vi "new recipe file - Copy.vi"() -> ()   [LabVIEW 2018]
uses:
  <vilib>/Utility/file.llb/Read Delimited Spreadsheet (string).vi
panel:
  out "error out 2":errorcluster caption="error out"
  out "error out":errorcluster
  in  "hidden tab":enum32{"Page 1"}(tab)
  out "L dc length step 20":string
  out "L dc length step 19":string
  out "L dc length step 18":string
  out "L dc length step 17":string
  out "L dc length step 16":string
  out "L dc length step 15":string
  out "L dc length step 14":string
  out "L dc length step 13":string
  out "L dc length step 12":string
  out "L dc length step 11":string
  out "L dc power step 20":string
  out "L dc power step 19":string
  out "L dc power step 18":string
  out "L dc power step 17":string
  out "L dc power step 16":string
  out "L dc power step 15":string
  out "L dc power step 14":string
  out "L dc power step 13":string
  out "L dc power step 12":string
  out "L dc power step 11":string
  out "L pressure":string
  out "L argon flow":string
  out "L rf length step 10":string
  out "L rf length step 9":string
  out "L rf length step 8":string
  out "L rf length step 7":string
  out "L rf length step 6":string
  out "L rf length step 5":string
  out "L rf length step 4":string
  out "L rf length step 3":string
  out "L rf length step 2":string
  out "L rf length step 1":string
  out "L rf power step 10":string
  out "L rf power step 9":string
  out "L rf power step 8":string
  out "L rf power step 7":string
  out "L rf power step 6":string
  out "L rf power step 5":string
  out "L rf power step 4":string
  out "L rf power step 3":string
  out "L rf power step 2":string
  out "L rf power step 1":string
  out "L dc length step 10":string
  out "L dc length step 9":string
  out "L dc length step 8":string
  out "L dc length step 7":string
  out "L dc length step 6":string
  out "L dc length step 5":string
  out "L dc length step 4":string
  out "L dc length step 3":string
  out "L dc length step 2":string
  out "L dc length step 1":string
  out "L dc power step 10":string
  out "L dc power step 9":string
  out "L dc power step 8":string
  out "L dc power step 7":string
  out "L dc power step 6":string
  out "L dc power step 5":string
  out "L dc power step 4":string
  out "L dc power step 3":string
  out "L dc power step 2":string
  out "L dc power step 1":string
  out "L microwave power":string
  out "L chamber selection":string
  out "L single process type selection":string
  out "L tension  value":string
  out "L web speed":string
  out "L web thickness":string
  out "L left init diamater":string
  out "L core diamater":string
  out "L web selection":string
  out "L recipe selection":string
  out "L sbs name":string
  out "L recipe name":string
  out "total length error":bool
  out "left diameter after roll":dbl=8.0
  out "done":bool
  out "L dc step number":string
  out "L rf step number":string
  out "L rf length step 11":string
  out "L rf length step 12":string
  out "L rf length step 13":string
  out "L rf length step 14":string
  out "L rf length step 15":string
  out "L rf length step 16":string
  out "L rf length step 17":string
  out "L rf length step 18":string
  out "L rf length step 19":string
  out "L rf length step 20":string
  out "L rf power step 11":string
  out "L rf power step 12":string
  out "L rf power step 13":string
  out "L rf power step 14":string
  out "L rf power step 15":string
  out "L rf power step 16":string
  out "L rf power step 17":string
  out "L rf power step 18":string
  out "L rf power step 19":string
  out "L rf power step 20":string
  in  "steplist tab RF":enum32{"Page 1", "Page 2"}(tab)
  in  "rf step watt 20":dbl
  in  "rf step watt 19":dbl
  in  "rf step watt 18":dbl
  in  "rf step watt 17":dbl
  in  "rf step watt 16":dbl
  in  "rf step watt 15":dbl
  in  "rf step watt 14":dbl
  in  "rf step watt 13":dbl
  in  "rf step watt 12":dbl
  in  "rf step watt 11":dbl
  in  "rf step length 20":dbl
  in  "rf step length 19":dbl
  in  "rf step length 18":dbl
  in  "rf step length 17":dbl
  in  "rf step length 16":dbl
  in  "rf step length 15":dbl
  in  "rf step length 14":dbl
  in  "rf step length 13":dbl
  in  "rf step length 12":dbl
  in  "rf step length 11":dbl
  in  "rf step length 1":dbl
  in  "rf step length 2":dbl
  in  "rf step length 3":dbl
  in  "rf step length 4":dbl
  in  "rf step length 5":dbl
  in  "rf step length 6":dbl
  in  "rf step length 7":dbl
  in  "rf step length 8":dbl
  in  "rf step length 9":dbl
  in  "rf step length 10":dbl
  in  "rf step watt 1":dbl
  in  "rf step watt 2":dbl
  in  "rf step watt 3":dbl
  in  "rf step watt 4":dbl
  in  "rf step watt 7":dbl
  in  "rf step watt 8":dbl
  in  "rf step watt 5":dbl
  in  "rf step watt 6":dbl
  in  "rf step watt 9":dbl
  in  "rf step watt 10":dbl
  in  "Step Number RF":u16(ring) items=["step 1"=1, "step 2"=2, "step 3"=3, "step 4"=4, "step 5"=5, "step 6"=6, "step 7"=7, "step 8"=8, "step 9"=9, "step 10"=10, "step 11"=11, "step 12"=12, "step 13"=13, "step 14"=14, "step 15"=15, "step 16"=16, "step 17"=17, "step 18"=18, "step 19"=19, "step 20"=20]
  out "concatenated string":string
  in  "steplist tab DC":enum32{"Page 1", "Page 2"}(tab)
  in  "dc step watt 1":dbl
  in  "dc step watt 2":dbl
  in  "dc step watt 3":dbl
  in  "dc step watt 4":dbl
  in  "dc step watt 5":dbl
  in  "dc step watt 6":dbl
  in  "dc step watt 7":dbl
  in  "dc step watt 8":dbl
  in  "dc step watt 9":dbl
  in  "dc step watt 10":dbl
  in  "dc step length 1":dbl
  in  "dc step length 2":dbl
  in  "dc step length 3":dbl
  in  "dc step length 4":dbl
  in  "dc step length 5":dbl
  in  "dc step length 6":dbl
  in  "dc step length 7":dbl
  in  "dc step length 8":dbl
  in  "dc step length 9":dbl
  in  "dc step length 10":dbl
  in  "Step Number DC":u16(ring) items=["step 1"=1, "step 2"=2, "step 3"=3, "step 4"=4, "step 5"=5, "step 6"=6, "step 7"=7, "step 8"=8, "step 9"=9, "step 10"=10, "step 11"=11, "step 12"=12, "step 13"=13, "step 14"=14, "step 15"=15, "step 16"=16, "step 17"=17, "step 18"=18, "step 19"=19, "step 20"=20]
  in  "dc step watt 20":dbl
  in  "dc step watt 19":dbl
  in  "dc step watt 18":dbl
  in  "dc step watt 17":dbl
  in  "dc step watt 16":dbl
  in  "dc step watt 15":dbl
  in  "dc step watt 14":dbl
  in  "dc step watt 13":dbl
  in  "dc step watt 12":dbl
  in  "dc step watt 11":dbl
  in  "dc step length 11":dbl
  in  "dc step length 12":dbl
  in  "dc step length 13":dbl
  in  "dc step length 14":dbl
  in  "dc step length 15":dbl
  in  "dc step length 16":dbl
  in  "dc step length 17":dbl
  in  "dc step length 18":dbl
  in  "dc step length 19":dbl
  in  "dc step length 20":dbl
  in  "General tab sub vi":enum32{"Page 1"}(tab)
  in  "Pressure set mbar":dbl=0.005 format="%#_1e"
  in  "Ar set sccm":dbl=20.0
  in  "CANCEL":bool
  in  "SAVE":bool
  in  "web-other tab":T1(tab)
  out "total length":dbl=500.0
  in  "tension value":dbl=7.0
  in  "web speed":dbl=250.0
  in  "web thickness":dbl=50.0
  in  "left initial diameter":dbl=94.0
  in  "core diameter":dbl=93.0
  in  "CALCULATE":bool
  in  "Web Selection":u16(ring) items=["web", "other"]
  in  "Recipe Selection":u16(ring) items=["single recipe", "multilayer recipe"]
  in  "Recipe Name":string
  in  "Substrate Material":string
  in  "recipe selection":T2(tab)
  in  "single process selection":enum32{"microwave", "dcsputter", "rfsputter"}(radio)
  in  "single process selection":T3(tab)
  in  "power microwave":dbl
  in  "DC Sputter Chamber Selection":enum32{"chamber II", "chamber III"}(radio)
  in  "power rf":dbl
  in  "web speed ch III ml":dbl=250.0
  in  "web speed ch II ml":dbl=250.0
  in  "LOAD":bool
  in  "password":bool
  in  "password":string
  # "Step List(RF)"
  # "power(watt)"
  # "length(cm)"
  # "Step 1"
  # "Step 2"
  # "Step 3"
  # "Step 4"
  # "Step 5"
  # "Step 6"
  # "Step 7"
  # "Step 8"
  # "Step 9"
  # "Step 10"
  # "Step 11"
  # "Step 12"
  # "Step 13"
  # "Step 14"
  # "Step 15"
  # "Step 16"
  # "Step 17"
  # "Step 18"
  # "Step 19"
  # "Step 20"
  # "Step List(DC)"
  # "power(watt)"
  # "length(cm)"
  # "Step 1"
  # "Step 2"
  # "Step 3"
  # "Step 4"
  # "Step 5"
  # "Step 6"
  # "Step 7"
  # "Step 8"
  # "Step 9"
  # "Step 10"
  # "Step 11"
  # "Step 12"
  # "Step 13"
  # "Step 14"
  # "Step 15"
  # "Step 16"
  # "Step 17"
  # "Step 18"
  # "Step 19"
  # "Step 20"
  # "Recipe Name"
  # "Subsrate Material"
  # "Recipe Selection"
  # "Web Selection"
  # "Argon Flow"
  # "sccm"
  # "Set Pressure"
  # "mbar"
  # "Core Diameter"
  # "mm"
  # "Web Speed"
  # "cm/min"
  # "Left InitialDiameter"
  # "mm"
  # "Tension Value"
  # "N"
  # "µm"
  # "cm"
  # "Web Thickness"
  # "Total Length"
  # "Power"
  # "watt"
  # "Power"
  # "watt"
  # "DCPS PARAMETERS"
  # "Chamber III"
  # "Chamber II"
  # "Web Speed"
  # "cm/min"
  # "Web Speed"
  # "cm/min"
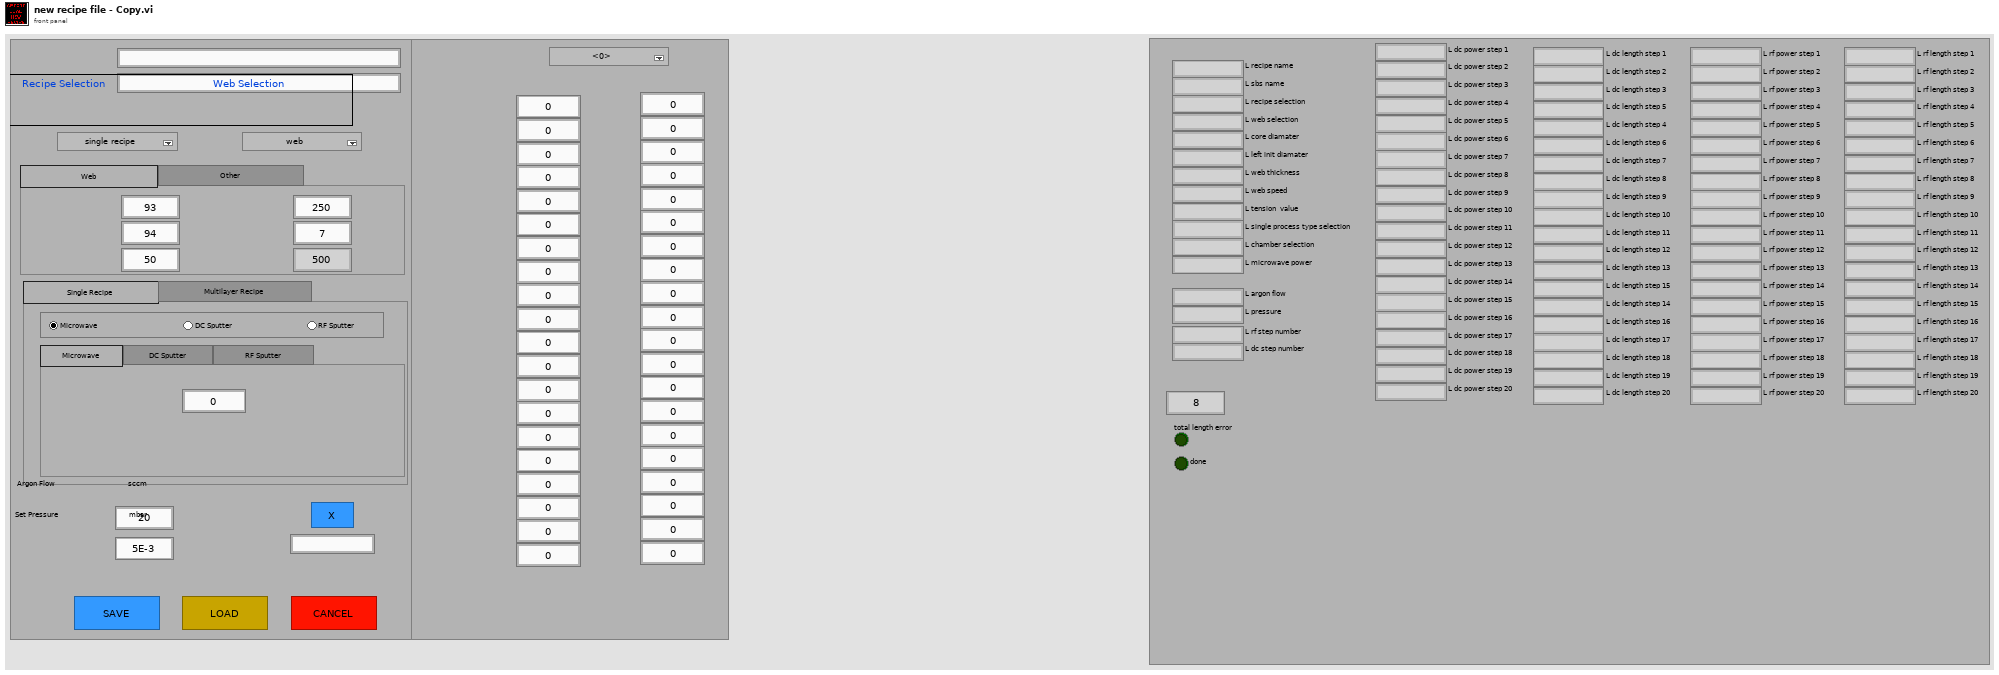
[diagram p1: front panel]
types:
  T1 = enum32{"Web                                                    ", "Other                                                      "}
  T2 = enum32{"Single Recipe                                    ", "Multilayer Recipe                                      "}
  T3 = enum32{"Microwave                ", "DC Sputter                   ", "RF Sputter                         "}
  T4 = enum16{"open", "replace", "create", "open or create", "replace or create", "replace or create with confirmation"}
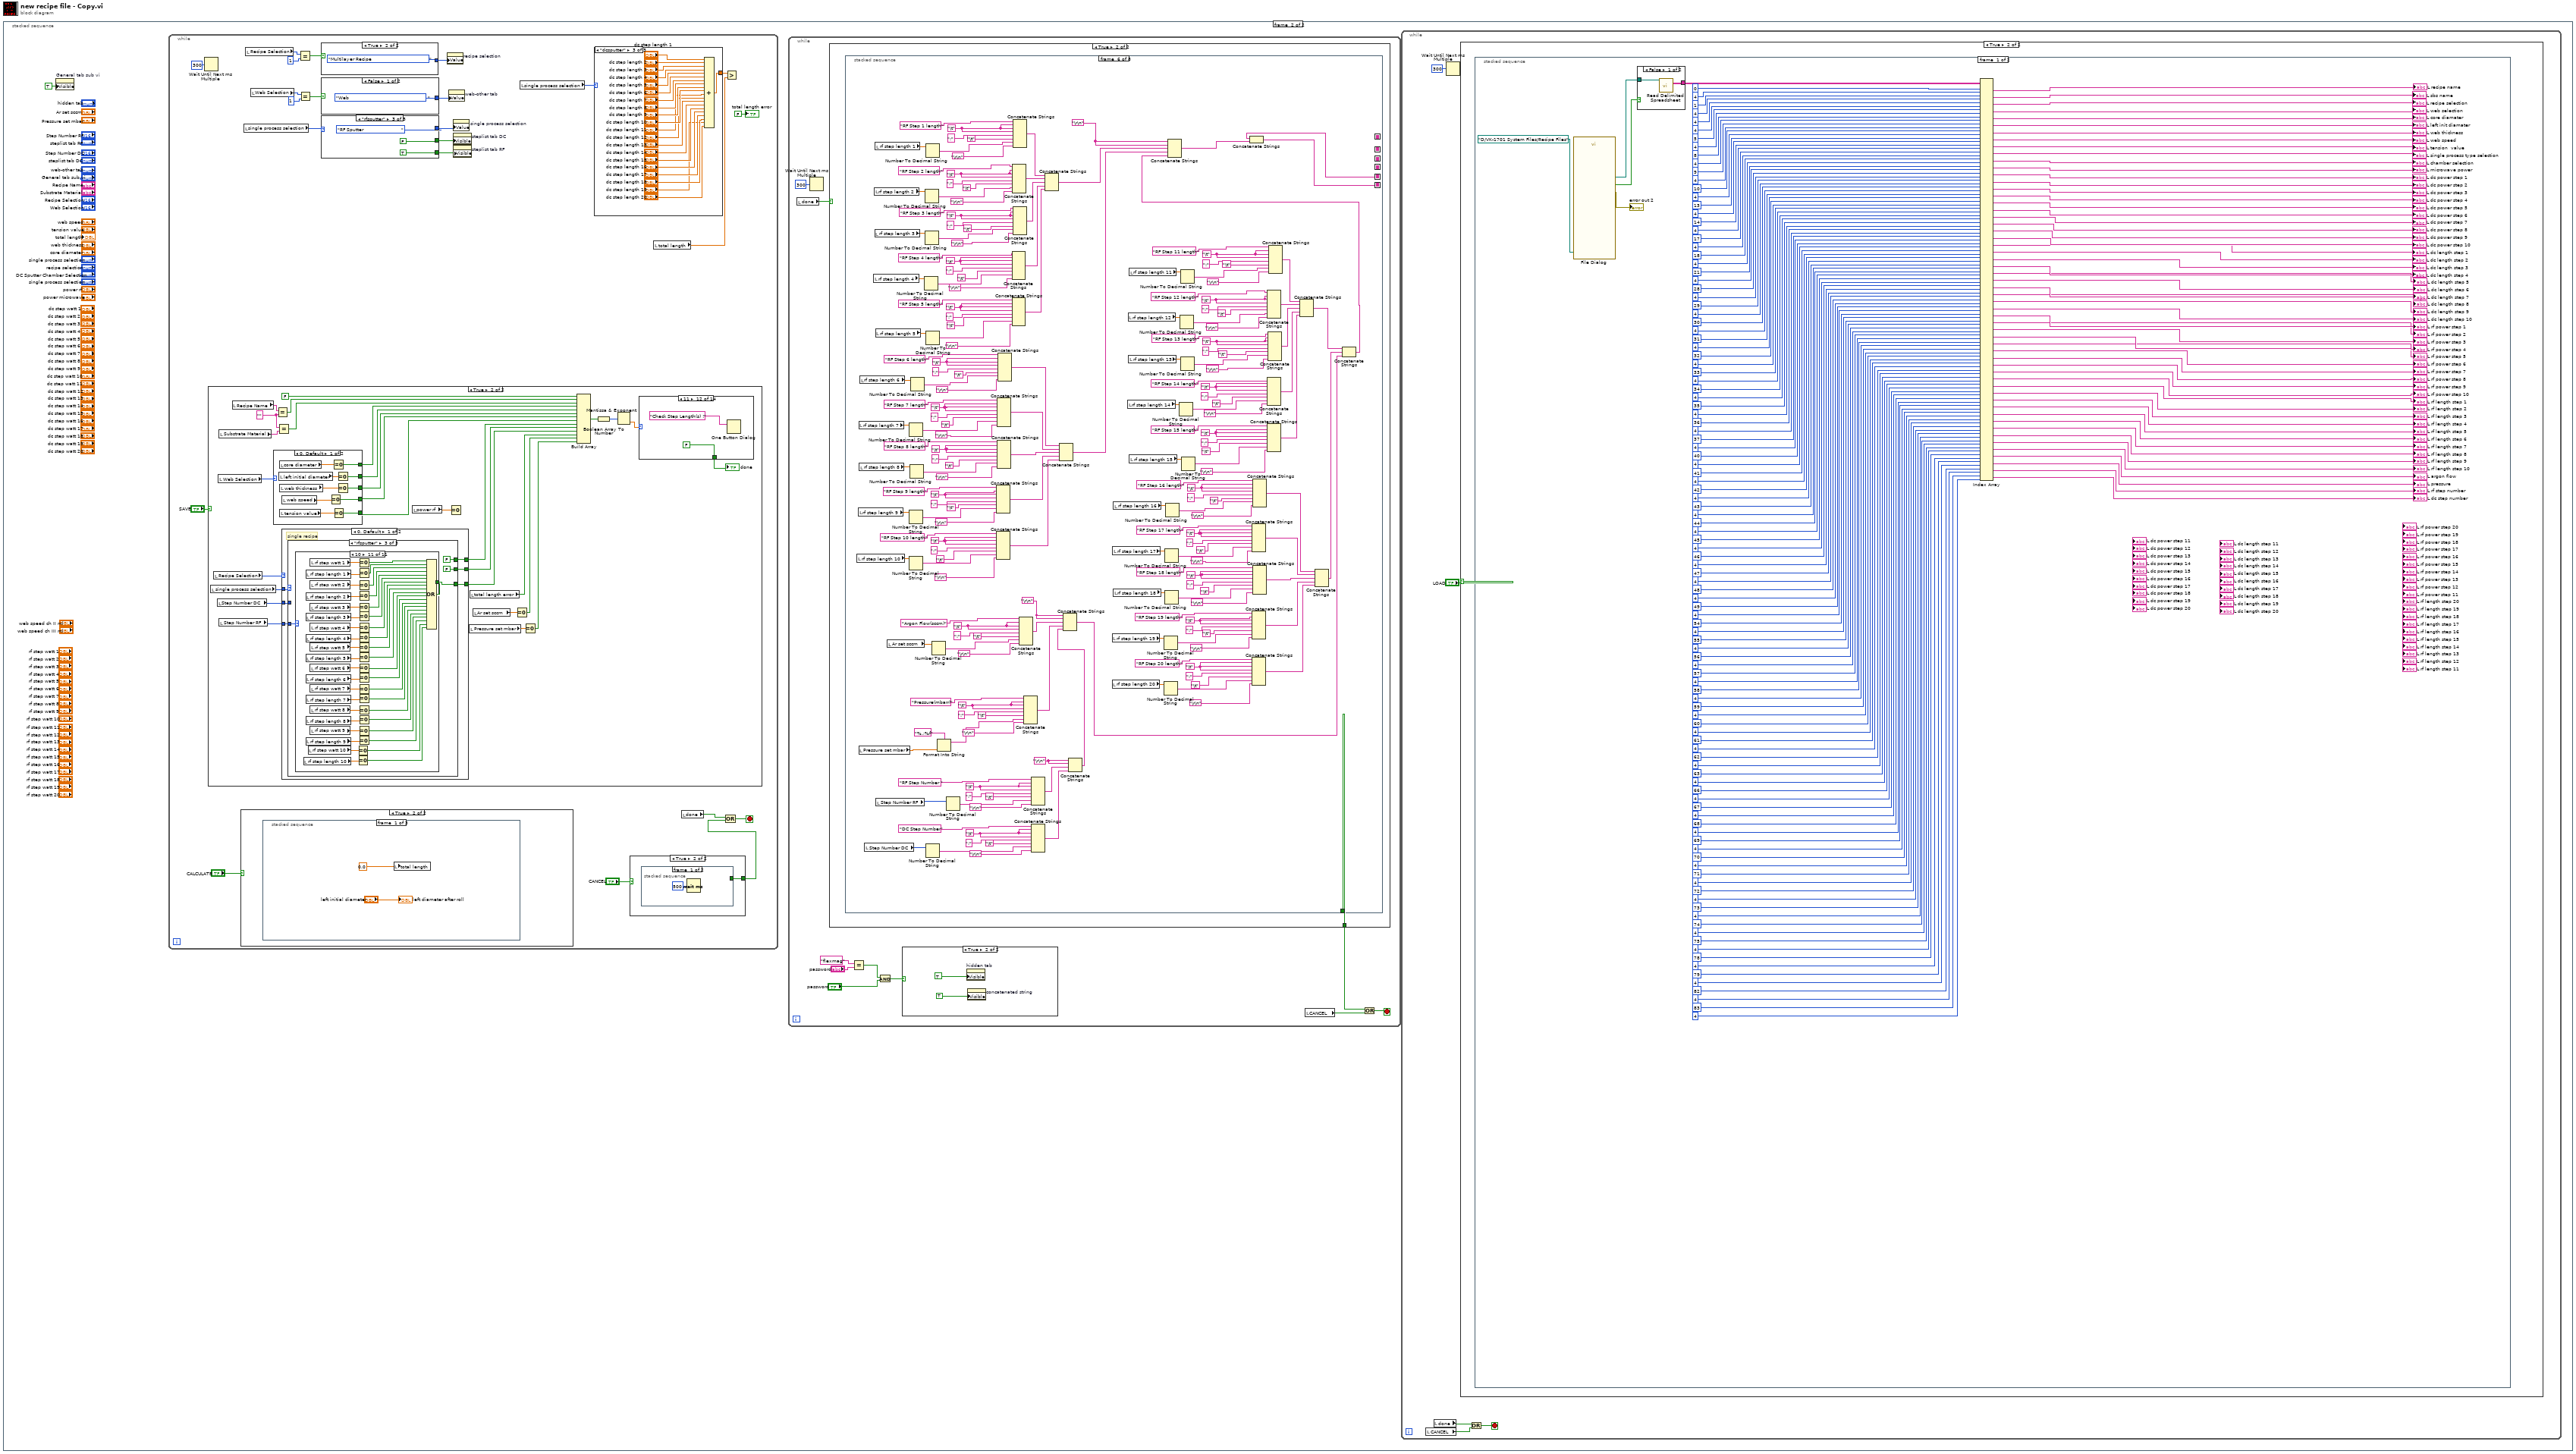
[diagram p0: block diagram]
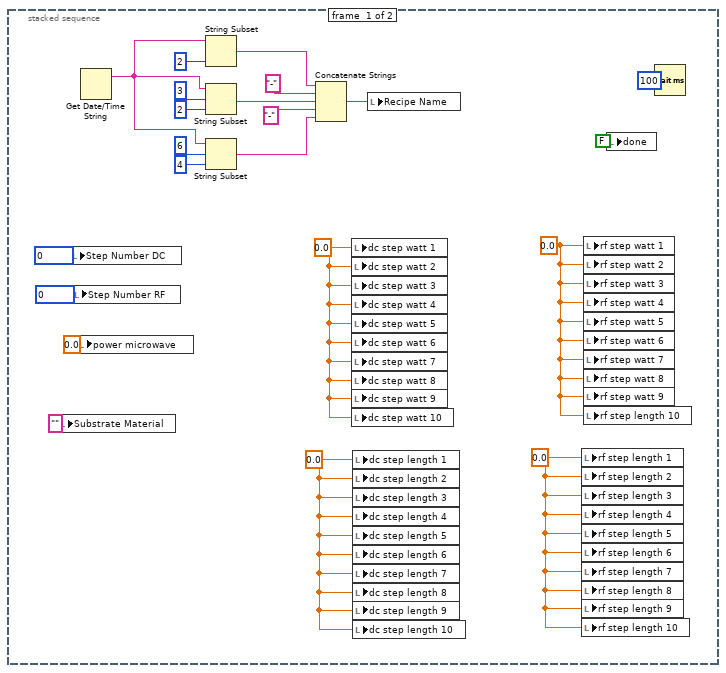
[diagram p2: hidden frame]
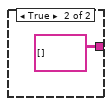
[diagram p4: hidden frame]
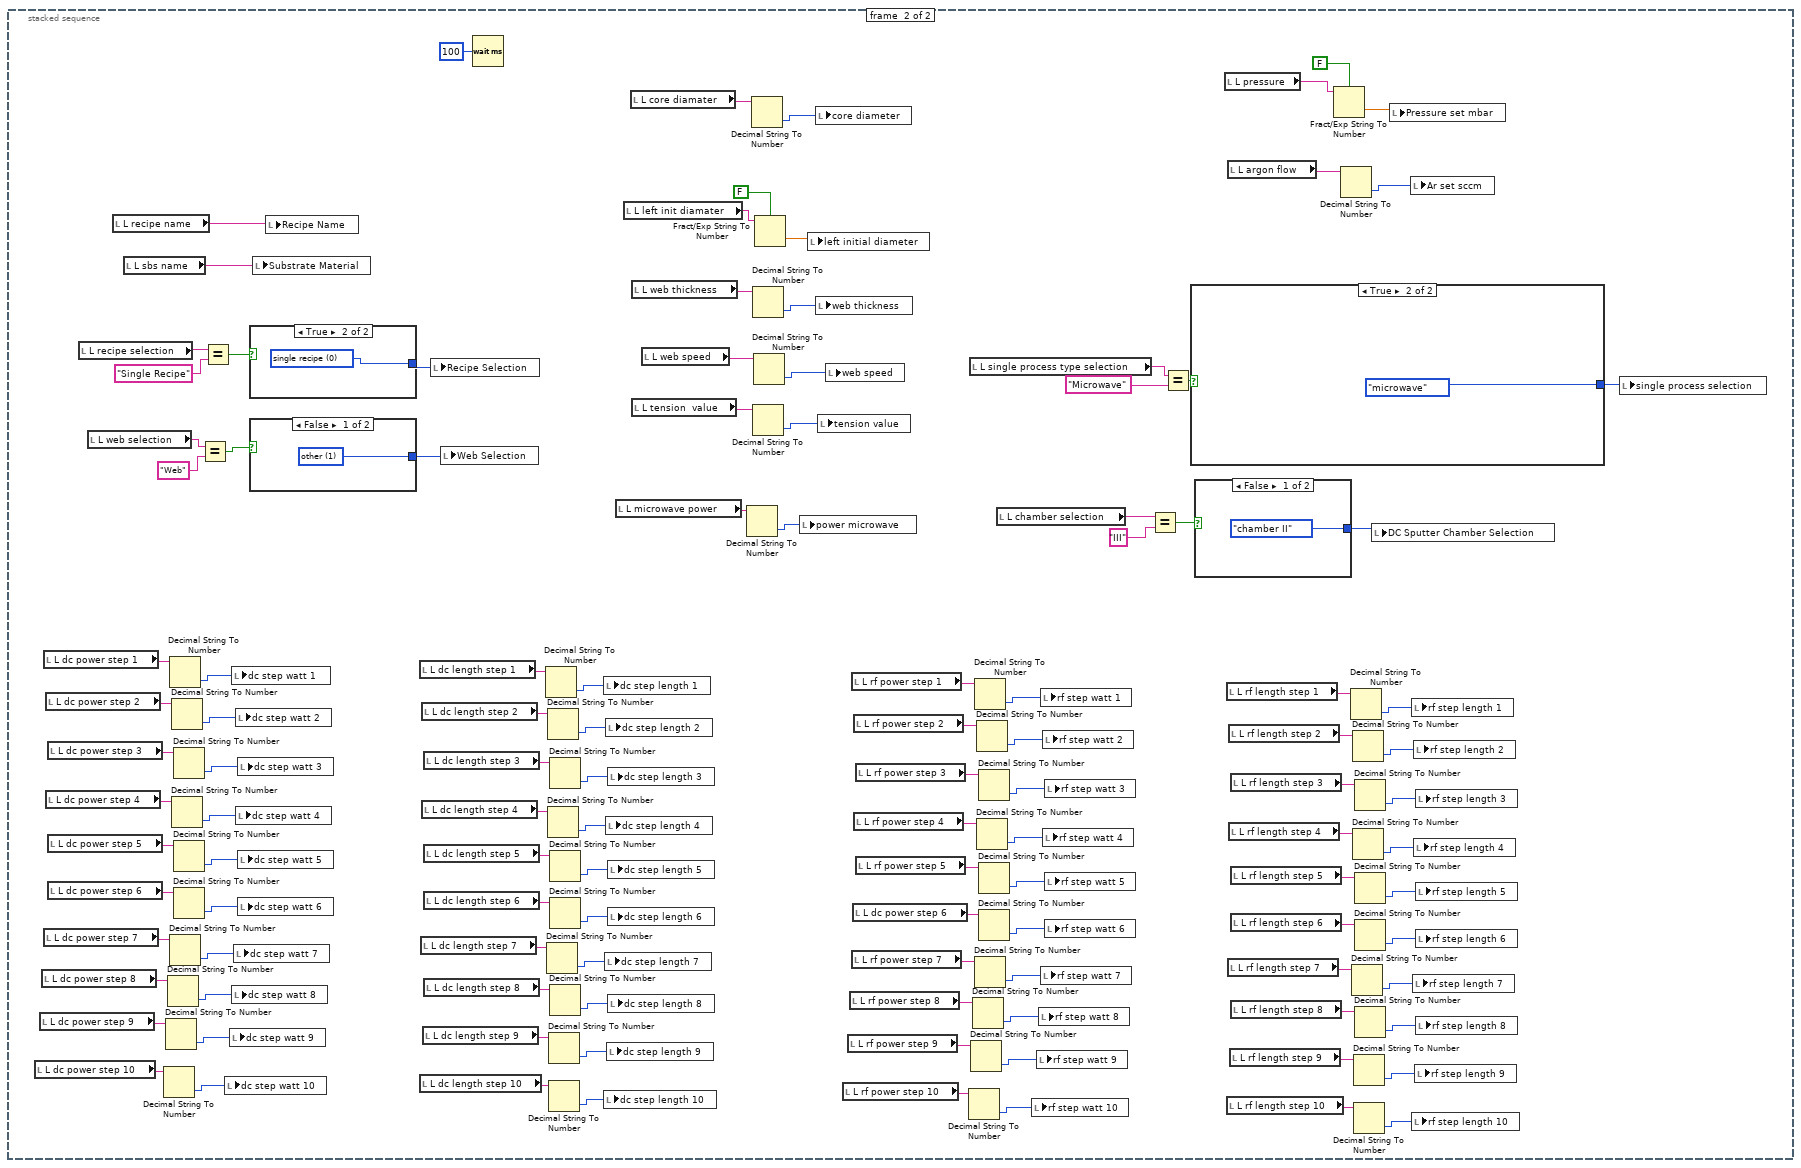
[diagram p5: hidden frame]
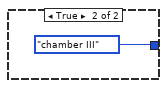
[diagram p6: hidden frame]
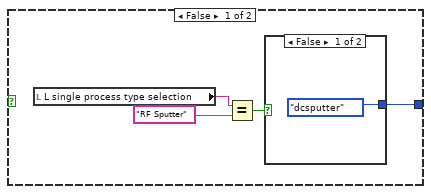
[diagram p7: hidden frame]
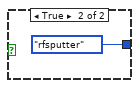
[diagram p8: hidden frame]
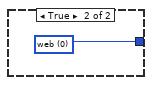
[diagram p9: hidden frame]
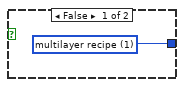
[diagram p10: hidden frame]
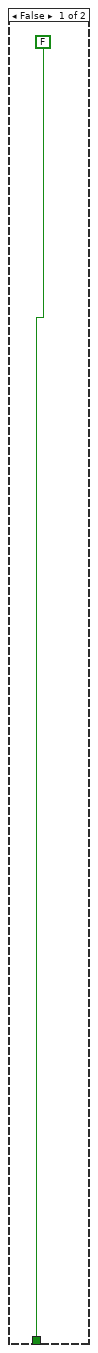
[diagram p12: hidden frame]
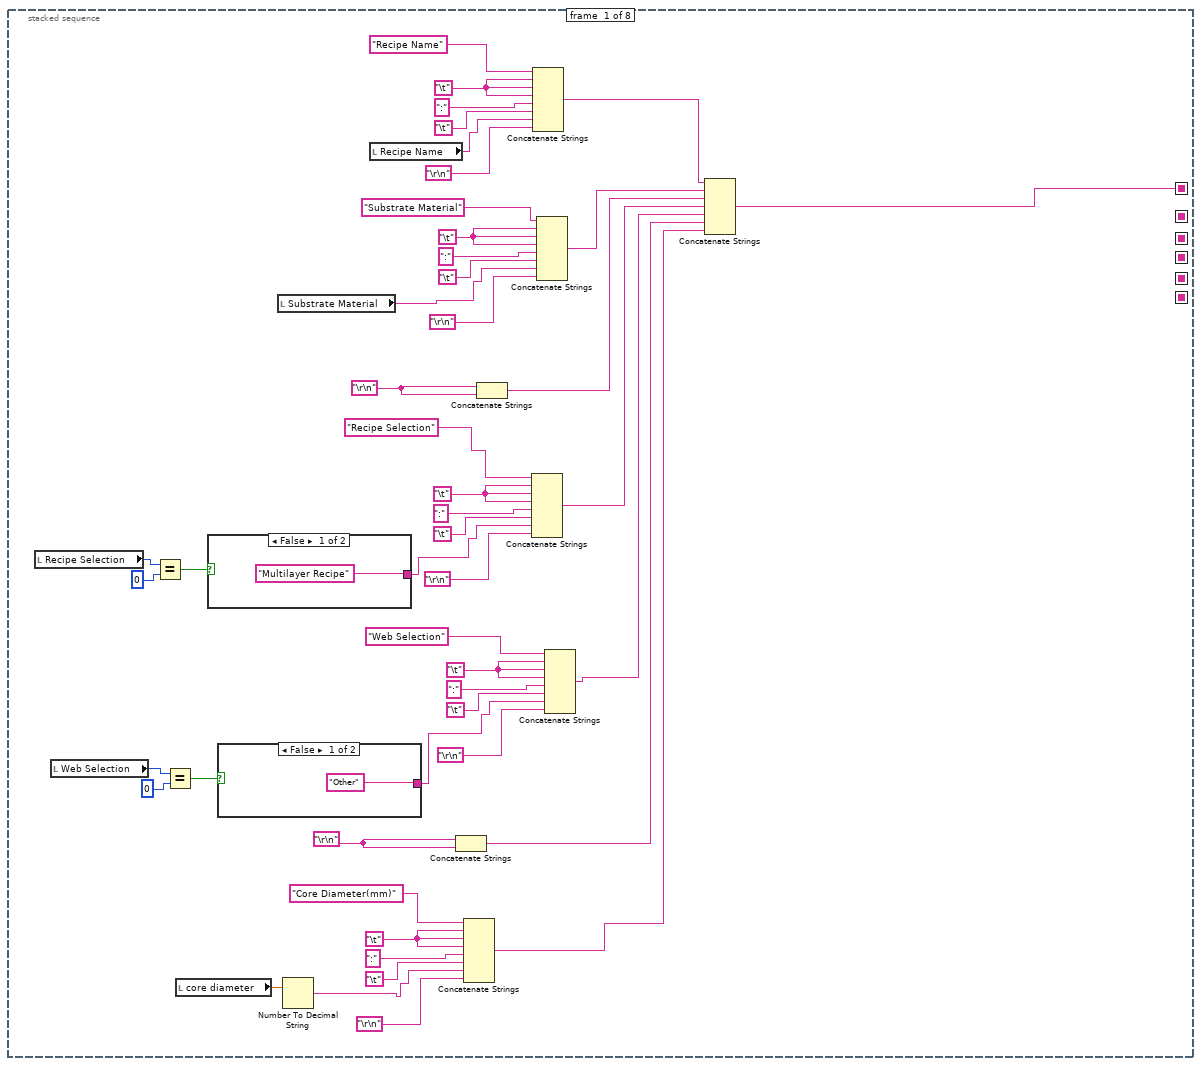
[diagram p13: hidden frame]
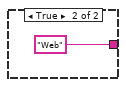
[diagram p14: hidden frame]
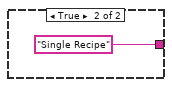
[diagram p15: hidden frame]
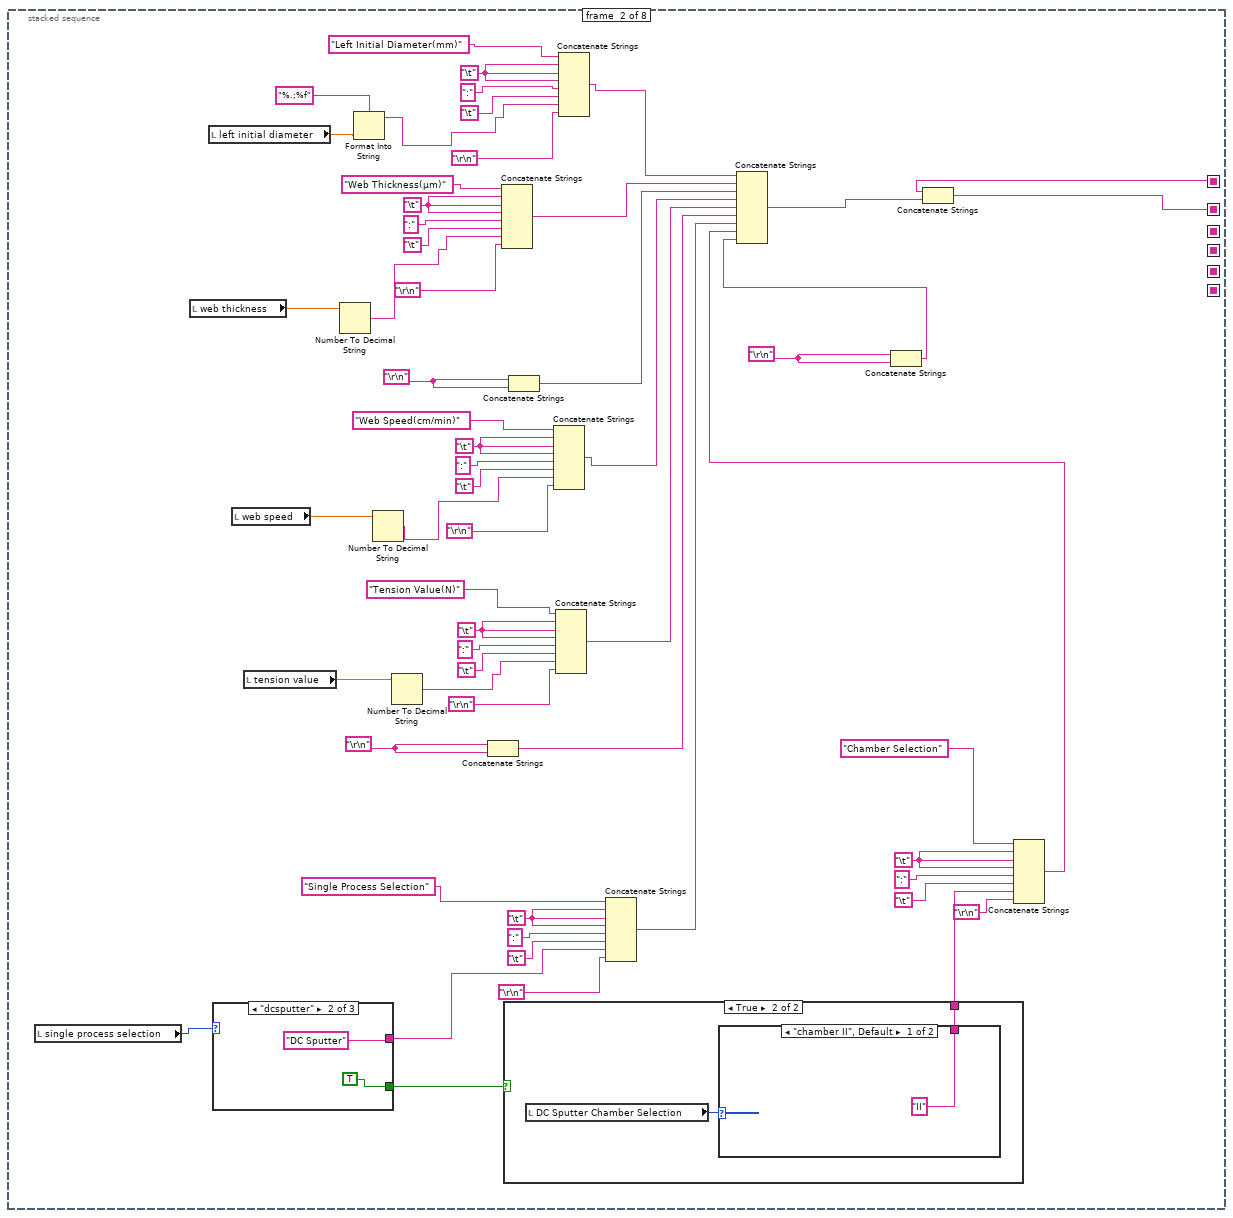
[diagram p16: hidden frame]
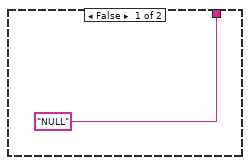
[diagram p17: hidden frame]
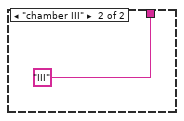
[diagram p18: hidden frame]
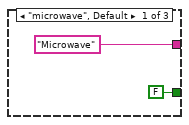
[diagram p19: hidden frame]
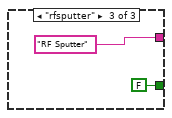
[diagram p20: hidden frame]
diagram:
  n1 = stacked-sequence {
    frame #0 {
      w3 = u16 0 items=["step 1"=1, "step 2"=2, "step 3"=3, "step 4"=4, "step 5"=5, "step 6"=6, "step 7"=7, "step 8"=8, "step 9"=9, "step 10"=10] ("Step Number DC")
      w5 = 0.0 ("dc step watt 1")
      w4 = 0.0 ("dc step watt 1")
      w6 = u16 0 items=["step 1"=1, "step 2"=2, "step 3"=3, "step 4"=4, "step 5"=5, "step 6"=6, "step 7"=7, "step 8"=8, "step 9"=9, "step 10"=10] ("Step Number DC")
      w7 = 0.0 ("dc step watt 1")
      w8 = 0.0 ("dc step watt 1")
      n2 = local write "Substrate Material"("" ("Substrate Material")) -> ()
      n3 = local write "Step Number DC"(w6) -> ()
      n4 = local write "Step Number RF"(w3) -> ()
      n5 = local write "power microwave"(0.0 ("power microwave")) -> ()
      n6 = Get Date/Time String() -> (date string=w16:string)  [unwired: 3 in, 1 out]
      n7 = String Subset(string=w16, length (rest)=2 ("length (rest)")) -> (substring=w17:string)  [unwired: 1 in]
      n8 = String Subset(string=w16, offset (0)=3, length (rest)=2 ("length (rest)")) -> (substring=w18:string)
      n9 = String Subset(string=w16, offset (0)=6, length (rest)=4 ("length (rest)")) -> (substring=w19:string)
      n10 = Concatenate Strings(w17, "-" ("string"), w18, "-" ("string"), w19) -> (w20:string)
      n11 = local write "dc step watt 1"(w8) -> ()
      n12 = local write "dc step watt 2"(w8) -> ()
      n13 = local write "dc step watt 3"(w8) -> ()
      n14 = local write "dc step watt 4"(w8) -> ()
      n15 = local write "dc step watt 5"(w8) -> ()
      n16 = local write "dc step watt 6"(w8) -> ()
      n17 = local write "dc step watt 7"(w8) -> ()
      n18 = local write "dc step watt 8"(w8) -> ()
      n19 = local write "dc step watt 9"(w8) -> ()
      n20 = local write "dc step watt 10"(w8) -> ()
      n21 = local write "dc step length 1"(w7) -> ()
      n22 = local write "dc step length 2"(w7) -> ()
      n23 = local write "dc step length 3"(w7) -> ()
      n24 = local write "dc step length 4"(w7) -> ()
      n25 = local write "dc step length 5"(w7) -> ()
      n26 = local write "dc step length 6"(w7) -> ()
      n27 = local write "dc step length 7"(w7) -> ()
      n28 = local write "dc step length 8"(w7) -> ()
      n29 = local write "dc step length 9"(w7) -> ()
      n30 = local write "dc step length 10"(w7) -> ()
      n31 = local write "Recipe Name"(w20) -> ()
      n32 = local write "rf step length 1"(w5) -> ()
      n33 = local write "rf step length 2"(w5) -> ()
      n34 = local write "rf step length 3"(w5) -> ()
      n35 = local write "rf step length 4"(w5) -> ()
      n36 = local write "rf step length 5"(w5) -> ()
      n37 = local write "rf step length 6"(w5) -> ()
      n38 = local write "rf step length 7"(w5) -> ()
      n39 = local write "rf step length 8"(w5) -> ()
      n40 = local write "rf step length 9"(w5) -> ()
      n41 = local write "rf step length 10"(w5) -> ()
      n42 = local write "rf step watt 1"(w4) -> ()
      n43 = local write "rf step watt 2"(w4) -> ()
      n44 = local write "rf step watt 3"(w4) -> ()
      n45 = local write "rf step watt 4"(w4) -> ()
      n46 = local write "rf step watt 5"(w4) -> ()
      n47 = local write "rf step watt 6"(w4) -> ()
      n48 = local write "rf step watt 7"(w4) -> ()
      n49 = local write "rf step watt 8"(w4) -> ()
      n50 = local write "rf step watt 9"(w4) -> ()
      n51 = local write "rf step length 10"(w4) -> ()
      n52 = local write "done"(FALSE ("done")) -> ()
      n53 = Wait (ms)(milliseconds to wait=u32 100) -> ()  [unwired: 1 out]
    }
    frame #1 {
      n54 = property on="General tab sub vi" class="TabCtl (strict)"("Visible"=TRUE) -> ()  [unwired: 2 in, 2 out]
      n55 = while {
        stop <- w1227 stop-if-true
        n56 = Wait Until Next ms Multiple(millisecond multiple=u32 300) -> ()  [unwired: 1 out]
        n57 = case shown="True" "SAVE" {
          frame False {
          }
          frame True {
            w1345 = "" ("y")
            n58 = local read "single process selection"() -> (w1331:enum32{"microwave", "dcsputter", "rfsputter"})
            n59 = local read "Recipe Selection"() -> (w1332:u16)
            n60 = local read "Step Number DC"() -> (w1330:u16)
            n61 = local read "Web Selection"() -> (w1339:u16)
            n62 = local read "Substrate Material"() -> (w1346:string)
            n63 = local read "Step Number RF"() -> (w1319:u16)
            n64 = local read "Recipe Name"() -> (w1347:string)
            n65 = case shown="0, Default" w1339 {
              tunnel: [w1836 w1841] -> w1338
              tunnel: [w1835 w1841] -> w1337
              tunnel: [w1834 w1841] -> w1336
              tunnel: [w1833 w1841] -> w1334
              tunnel: [w1831 w1841] -> w1335
              frame 0, Default {
                n66 = local read "left initial diameter"() -> (w1839:dbl)
                n67 = local read "core diameter"() -> (w1840:dbl)
                n68 = local read "web thickness"() -> (w1838:dbl)
                n69 = local read "tension value"() -> (w1837:dbl)
                n70 = local read "web speed"() -> (w1832:dbl)
                n71 = Equal To 0?(x=w1832) -> (x = 0?=w1831:bool)
                n72 = Equal To 0?(x=w1840) -> (x = 0?=w1836:bool)
                n73 = Equal To 0?(x=w1837) -> (x = 0?=w1833:bool)
                n74 = Equal To 0?(x=w1839) -> (x = 0?=w1835:bool)
                n75 = Equal To 0?(x=w1838) -> (x = 0?=w1834:bool)
              }
              frame 1 {
                w1841 = FALSE
              }
            }
            n76 = Equal?(x=w1347, y=w1345) -> (x = y?=w1341:bool)
            n77 = Equal?(x=w1345, y=w1346) -> (x = y?=w1340:bool)
            n78 = case shown="0, Default" w1332 {
              tunnel: w1331 -> [w1353 _]
              tunnel: w1330 -> [w1352 _]
              tunnel: [w1351 FALSE] -> w1329
              tunnel: [w1350 FALSE] -> w1328
              tunnel: [w1349 FALSE] -> w1327
              tunnel: w1319 -> [w1348 _]
              frame 0, Default {
                # "single recipe"
                n79 = case shown="\"rfsputter\"" w1353 {
                  tunnel: w1352 -> [_ w1361 _]
                  tunnel: [w1356 FALSE FALSE] -> w1351
                  tunnel: [FALSE w1360 FALSE] -> w1350
                  tunnel: [FALSE FALSE w1594] -> w1349
                  tunnel: w1348 -> [_ _ w1593]
                  frame "microwave", Default {
                    n80 = local read "power microwave"() -> (w1357:dbl)
                    n81 = Equal To 0?(x=w1357) -> (x = 0?=w1356:bool)
                  }
                  frame "dcsputter" {
                    n82 = case shown="1" w1361 {
                      tunnel: [FALSE w1363 w1372 w1385 w1402 w1423 w1448 w1477 w1510 w1547 w1588] -> w1360
                      frame 0, Default {
                      }
                      frame 1 {
                        n83 = local read "dc step length 1"() -> (w1366:dbl)
                        n84 = local read "dc step watt 1"() -> (w1367:dbl)
                        n85 = Equal To 0?(x=w1367) -> (x = 0?=w1365:bool)
                        n86 = Equal To 0?(x=w1366) -> (x = 0?=w1364:bool)
                        n87 = Compound Arithmetic op=OR(w1365, w1364) -> (w1363:bool)
                      }
                      frame 2 {
                        n88 = local read "dc step length 1"() -> (w1375:dbl)
                        n89 = local read "dc step length 2"() -> (w1371:dbl)
                        n90 = local read "dc step watt 1"() -> (w1376:dbl)
                        n91 = local read "dc step watt 2"() -> (w1370:dbl)
                        n92 = Equal To 0?(x=w1376) -> (x = 0?=w1374:bool)
                        n93 = Equal To 0?(x=w1370) -> (x = 0?=w1369:bool)
                        n94 = Equal To 0?(x=w1375) -> (x = 0?=w1373:bool)
                        n95 = Equal To 0?(x=w1371) -> (x = 0?=w1368:bool)
                        n96 = Compound Arithmetic op=OR(w1374, w1373, w1369, w1368) -> (w1372:bool)
                      }
                      frame 3 {
                        n97 = local read "dc step length 1"() -> (w1388:dbl)
                        n98 = local read "dc step length 2"() -> (w1384:dbl)
                        n99 = local read "dc step length 3"() -> (w1379:dbl)
                        n100 = local read "dc step watt 1"() -> (w1389:dbl)
                        n101 = local read "dc step watt 2"() -> (w1383:dbl)
                        n102 = local read "dc step watt 3"() -> (w1380:dbl)
                        n103 = Equal To 0?(x=w1389) -> (x = 0?=w1387:bool)
                        n104 = Equal To 0?(x=w1383) -> (x = 0?=w1382:bool)
                        n105 = Equal To 0?(x=w1388) -> (x = 0?=w1386:bool)
                        n106 = Equal To 0?(x=w1380) -> (x = 0?=w1378:bool)
                        n107 = Equal To 0?(x=w1384) -> (x = 0?=w1381:bool)
                        n108 = Equal To 0?(x=w1379) -> (x = 0?=w1377:bool)
                        n109 = Compound Arithmetic op=OR(w1387, w1386, w1382, w1381, w1378, w1377) -> (w1385:bool)
                      }
                      frame 4 {
                        n110 = local read "dc step length 1"() -> (w1405:dbl)
                        n111 = local read "dc step length 4"() -> (w1393:dbl)
                        n112 = local read "dc step length 2"() -> (w1401:dbl)
                        n113 = local read "dc step length 3"() -> (w1396:dbl)
                        n114 = local read "dc step watt 1"() -> (w1406:dbl)
                        n115 = local read "dc step watt 2"() -> (w1400:dbl)
                        n116 = local read "dc step watt 4"() -> (w1392:dbl)
                        n117 = local read "dc step watt 3"() -> (w1397:dbl)
                        n118 = Equal To 0?(x=w1406) -> (x = 0?=w1404:bool)
                        n119 = Equal To 0?(x=w1400) -> (x = 0?=w1399:bool)
                        n120 = Equal To 0?(x=w1392) -> (x = 0?=w1391:bool)
                        n121 = Equal To 0?(x=w1405) -> (x = 0?=w1403:bool)
                        n122 = Equal To 0?(x=w1397) -> (x = 0?=w1395:bool)
                        n123 = Equal To 0?(x=w1393) -> (x = 0?=w1390:bool)
                        n124 = Equal To 0?(x=w1401) -> (x = 0?=w1398:bool)
                        n125 = Equal To 0?(x=w1396) -> (x = 0?=w1394:bool)
                        n126 = Compound Arithmetic op=OR(w1404, w1403, w1399, w1398, w1395, w1394, w1391, w1390) -> (w1402:bool)
                      }
                      frame 5 {
                        n127 = local read "dc step length 5"() -> (w1409:dbl)
                        n128 = local read "dc step length 1"() -> (w1426:dbl)
                        n129 = local read "dc step length 4"() -> (w1414:dbl)
                        n130 = local read "dc step length 2"() -> (w1422:dbl)
                        n131 = local read "dc step length 3"() -> (w1417:dbl)
                        n132 = local read "dc step watt 1"() -> (w1427:dbl)
                        n133 = local read "dc step watt 5"() -> (w1410:dbl)
                        n134 = local read "dc step watt 2"() -> (w1421:dbl)
                        n135 = local read "dc step watt 4"() -> (w1413:dbl)
                        n136 = local read "dc step watt 3"() -> (w1418:dbl)
                        n137 = Equal To 0?(x=w1410) -> (x = 0?=w1408:bool)
                        n138 = Equal To 0?(x=w1427) -> (x = 0?=w1425:bool)
                        n139 = Equal To 0?(x=w1409) -> (x = 0?=w1407:bool)
                        n140 = Equal To 0?(x=w1421) -> (x = 0?=w1420:bool)
                        n141 = Equal To 0?(x=w1413) -> (x = 0?=w1412:bool)
                        n142 = Equal To 0?(x=w1426) -> (x = 0?=w1424:bool)
                        n143 = Equal To 0?(x=w1418) -> (x = 0?=w1416:bool)
                        n144 = Equal To 0?(x=w1414) -> (x = 0?=w1411:bool)
                        n145 = Equal To 0?(x=w1422) -> (x = 0?=w1419:bool)
                        n146 = Equal To 0?(x=w1417) -> (x = 0?=w1415:bool)
                        n147 = Compound Arithmetic op=OR(w1425, w1424, w1420, w1419, w1416, w1415, w1412, w1411, w1408, w1407) -> (w1423:bool)
                      }
                      frame 6 {
                        n148 = local read "dc step length 6"() -> (w1431:dbl)
                        n149 = local read "dc step length 5"() -> (w1434:dbl)
                        n150 = local read "dc step length 1"() -> (w1451:dbl)
                        n151 = local read "dc step length 4"() -> (w1439:dbl)
                        n152 = local read "dc step length 2"() -> (w1447:dbl)
                        n153 = local read "dc step length 3"() -> (w1442:dbl)
                        n154 = local read "dc step watt 6"() -> (w1430:dbl)
                        n155 = local read "dc step watt 1"() -> (w1452:dbl)
                        n156 = local read "dc step watt 5"() -> (w1435:dbl)
                        n157 = local read "dc step watt 2"() -> (w1446:dbl)
                        n158 = local read "dc step watt 4"() -> (w1438:dbl)
                        n159 = local read "dc step watt 3"() -> (w1443:dbl)
                        n160 = Equal To 0?(x=w1430) -> (x = 0?=w1429:bool)
                        n161 = Equal To 0?(x=w1431) -> (x = 0?=w1428:bool)
                        n162 = Equal To 0?(x=w1435) -> (x = 0?=w1433:bool)
                        n163 = Equal To 0?(x=w1452) -> (x = 0?=w1450:bool)
                        n164 = Equal To 0?(x=w1434) -> (x = 0?=w1432:bool)
                        n165 = Equal To 0?(x=w1446) -> (x = 0?=w1445:bool)
                        n166 = Equal To 0?(x=w1438) -> (x = 0?=w1437:bool)
                        n167 = Equal To 0?(x=w1451) -> (x = 0?=w1449:bool)
                        n168 = Equal To 0?(x=w1443) -> (x = 0?=w1441:bool)
                        n169 = Equal To 0?(x=w1439) -> (x = 0?=w1436:bool)
                        n170 = Equal To 0?(x=w1447) -> (x = 0?=w1444:bool)
                        n171 = Equal To 0?(x=w1442) -> (x = 0?=w1440:bool)
                        n172 = Compound Arithmetic op=OR(w1450, w1449, w1445, w1444, w1441, w1440, w1437, w1436, w1433, w1432, w1429, w1428) -> (w1448:bool)
                      }
                      frame 7 {
                        n173 = local read "dc step length 6"() -> (w1460:dbl)
                        n174 = local read "dc step length 7"() -> (w1455:dbl)
                        n175 = local read "dc step length 5"() -> (w1463:dbl)
                        n176 = local read "dc step length 1"() -> (w1480:dbl)
                        n177 = local read "dc step length 4"() -> (w1468:dbl)
                        n178 = local read "dc step length 2"() -> (w1476:dbl)
                        n179 = local read "dc step length 3"() -> (w1471:dbl)
                        n180 = local read "dc step watt 6"() -> (w1459:dbl)
                        n181 = local read "dc step watt 7"() -> (w1456:dbl)
                        n182 = local read "dc step watt 1"() -> (w1481:dbl)
                        n183 = local read "dc step watt 5"() -> (w1464:dbl)
                        n184 = local read "dc step watt 2"() -> (w1475:dbl)
                        n185 = local read "dc step watt 4"() -> (w1467:dbl)
                        n186 = local read "dc step watt 3"() -> (w1472:dbl)
                        n187 = Equal To 0?(x=w1459) -> (x = 0?=w1458:bool)
                        n188 = Equal To 0?(x=w1456) -> (x = 0?=w1454:bool)
                        n189 = Equal To 0?(x=w1460) -> (x = 0?=w1457:bool)
                        n190 = Equal To 0?(x=w1455) -> (x = 0?=w1453:bool)
                        n191 = Equal To 0?(x=w1464) -> (x = 0?=w1462:bool)
                        n192 = Equal To 0?(x=w1481) -> (x = 0?=w1479:bool)
                        n193 = Equal To 0?(x=w1463) -> (x = 0?=w1461:bool)
                        n194 = Equal To 0?(x=w1475) -> (x = 0?=w1474:bool)
                        n195 = Equal To 0?(x=w1467) -> (x = 0?=w1466:bool)
                        n196 = Equal To 0?(x=w1480) -> (x = 0?=w1478:bool)
                        n197 = Equal To 0?(x=w1472) -> (x = 0?=w1470:bool)
                        n198 = Equal To 0?(x=w1468) -> (x = 0?=w1465:bool)
                        n199 = Equal To 0?(x=w1476) -> (x = 0?=w1473:bool)
                        n200 = Equal To 0?(x=w1471) -> (x = 0?=w1469:bool)
                        n201 = Compound Arithmetic op=OR(w1479, w1478, w1474, w1473, w1470, w1469, w1466, w1465, w1462, w1461, w1458, w1457, w1454, w1453) -> (w1477:bool)
                      }
                      frame 8 {
                        n202 = local read "dc step length 6"() -> (w1493:dbl)
                        n203 = local read "dc step length 7"() -> (w1488:dbl)
                        n204 = local read "dc step length 8"() -> (w1485:dbl)
                        n205 = local read "dc step length 5"() -> (w1496:dbl)
                        n206 = local read "dc step length 1"() -> (w1513:dbl)
                        n207 = local read "dc step length 4"() -> (w1501:dbl)
                        n208 = local read "dc step length 2"() -> (w1509:dbl)
                        n209 = local read "dc step length 3"() -> (w1504:dbl)
                        n210 = local read "dc step watt 6"() -> (w1492:dbl)
                        n211 = local read "dc step watt 7"() -> (w1489:dbl)
                        n212 = local read "dc step watt 8"() -> (w1484:dbl)
                        n213 = local read "dc step watt 1"() -> (w1514:dbl)
                        n214 = local read "dc step watt 5"() -> (w1497:dbl)
                        n215 = local read "dc step watt 2"() -> (w1508:dbl)
                        n216 = local read "dc step watt 4"() -> (w1500:dbl)
                        n217 = local read "dc step watt 3"() -> (w1505:dbl)
                        n218 = Equal To 0?(x=w1492) -> (x = 0?=w1491:bool)
                        n219 = Equal To 0?(x=w1489) -> (x = 0?=w1487:bool)
                        n220 = Equal To 0?(x=w1493) -> (x = 0?=w1490:bool)
                        n221 = Equal To 0?(x=w1488) -> (x = 0?=w1486:bool)
                        n222 = Equal To 0?(x=w1484) -> (x = 0?=w1483:bool)
                        n223 = Equal To 0?(x=w1497) -> (x = 0?=w1495:bool)
                        n224 = Equal To 0?(x=w1485) -> (x = 0?=w1482:bool)
                        n225 = Equal To 0?(x=w1514) -> (x = 0?=w1512:bool)
                        n226 = Equal To 0?(x=w1496) -> (x = 0?=w1494:bool)
                        n227 = Equal To 0?(x=w1508) -> (x = 0?=w1507:bool)
                        n228 = Equal To 0?(x=w1500) -> (x = 0?=w1499:bool)
                        n229 = Equal To 0?(x=w1513) -> (x = 0?=w1511:bool)
                        n230 = Equal To 0?(x=w1505) -> (x = 0?=w1503:bool)
                        n231 = Equal To 0?(x=w1501) -> (x = 0?=w1498:bool)
                        n232 = Equal To 0?(x=w1509) -> (x = 0?=w1506:bool)
                        n233 = Equal To 0?(x=w1504) -> (x = 0?=w1502:bool)
                        n234 = Compound Arithmetic op=OR(w1512, w1511, w1507, w1506, w1503, w1502, w1499, w1498, w1495, w1494, w1491, w1490, w1487, w1486, w1483, w1482) -> (w1510:bool)
                      }
                      frame 9 {
                        n235 = local read "dc step length 1"() -> (w1550:dbl)
                        n236 = local read "dc step length 2"() -> (w1546:dbl)
                        n237 = local read "dc step length 3"() -> (w1541:dbl)
                        n238 = local read "dc step length 4"() -> (w1538:dbl)
                        n239 = local read "dc step length 5"() -> (w1533:dbl)
                        n240 = local read "dc step length 6"() -> (w1530:dbl)
                        n241 = local read "dc step length 7"() -> (w1525:dbl)
                        n242 = local read "dc step length 8"() -> (w1522:dbl)
                        n243 = local read "dc step length 9"() -> (w1517:dbl)
                        n244 = local read "dc step watt 1"() -> (w1551:dbl)
                        n245 = local read "dc step watt 2"() -> (w1545:dbl)
                        n246 = local read "dc step watt 3"() -> (w1542:dbl)
                        n247 = local read "dc step watt 4"() -> (w1537:dbl)
                        n248 = local read "dc step watt 5"() -> (w1534:dbl)
                        n249 = local read "dc step watt 6"() -> (w1529:dbl)
                        n250 = local read "dc step watt 7"() -> (w1526:dbl)
                        n251 = local read "dc step watt 8"() -> (w1521:dbl)
                        n252 = local read "dc step watt 9"() -> (w1518:dbl)
                        n253 = Equal To 0?(x=w1529) -> (x = 0?=w1528:bool)
                        n254 = Equal To 0?(x=w1526) -> (x = 0?=w1524:bool)
                        n255 = Equal To 0?(x=w1530) -> (x = 0?=w1527:bool)
                        n256 = Equal To 0?(x=w1525) -> (x = 0?=w1523:bool)
                        n257 = Equal To 0?(x=w1521) -> (x = 0?=w1520:bool)
                        n258 = Equal To 0?(x=w1534) -> (x = 0?=w1532:bool)
                        n259 = Equal To 0?(x=w1522) -> (x = 0?=w1519:bool)
                        n260 = Equal To 0?(x=w1551) -> (x = 0?=w1549:bool)
                        n261 = Equal To 0?(x=w1533) -> (x = 0?=w1531:bool)
                        n262 = Equal To 0?(x=w1545) -> (x = 0?=w1544:bool)
                        n263 = Equal To 0?(x=w1537) -> (x = 0?=w1536:bool)
                        n264 = Equal To 0?(x=w1518) -> (x = 0?=w1516:bool)
                        n265 = Equal To 0?(x=w1550) -> (x = 0?=w1548:bool)
                        n266 = Equal To 0?(x=w1542) -> (x = 0?=w1540:bool)
                        n267 = Equal To 0?(x=w1538) -> (x = 0?=w1535:bool)
                        n268 = Equal To 0?(x=w1546) -> (x = 0?=w1543:bool)
                        n269 = Equal To 0?(x=w1541) -> (x = 0?=w1539:bool)
                        n270 = Equal To 0?(x=w1517) -> (x = 0?=w1515:bool)
                        n271 = Compound Arithmetic op=OR(w1549, w1548, w1544, w1543, w1540, w1539, w1536, w1535, w1532, w1531, w1528, w1527, w1524, w1523, w1520, w1519, w1516, w1515) -> (w1547:bool)
                      }
                      frame 10 {
                        n272 = local read "dc step length 10"() -> (w1555:dbl)
                        n273 = local read "dc step length 1"() -> (w1591:dbl)
                        n274 = local read "dc step length 2"() -> (w1587:dbl)
                        n275 = local read "dc step length 3"() -> (w1582:dbl)
                        n276 = local read "dc step length 4"() -> (w1579:dbl)
                        n277 = local read "dc step length 5"() -> (w1574:dbl)
                        n278 = local read "dc step length 6"() -> (w1571:dbl)
                        n279 = local read "dc step length 7"() -> (w1566:dbl)
                        n280 = local read "dc step length 8"() -> (w1563:dbl)
                        n281 = local read "dc step length 9"() -> (w1558:dbl)
                        n282 = local read "dc step watt 10"() -> (w1554:dbl)
                        n283 = local read "dc step watt 1"() -> (w1592:dbl)
                        n284 = local read "dc step watt 2"() -> (w1586:dbl)
                        n285 = local read "dc step watt 3"() -> (w1583:dbl)
                        n286 = local read "dc step watt 4"() -> (w1578:dbl)
                        n287 = local read "dc step watt 5"() -> (w1575:dbl)
                        n288 = local read "dc step watt 6"() -> (w1570:dbl)
                        n289 = local read "dc step watt 7"() -> (w1567:dbl)
                        n290 = local read "dc step watt 8"() -> (w1562:dbl)
                        n291 = local read "dc step watt 9"() -> (w1559:dbl)
                        n292 = Equal To 0?(x=w1592) -> (x = 0?=w1590:bool)
                        n293 = Equal To 0?(x=w1591) -> (x = 0?=w1589:bool)
                        n294 = Equal To 0?(x=w1586) -> (x = 0?=w1585:bool)
                        n295 = Equal To 0?(x=w1587) -> (x = 0?=w1584:bool)
                        n296 = Equal To 0?(x=w1583) -> (x = 0?=w1581:bool)
                        n297 = Equal To 0?(x=w1582) -> (x = 0?=w1580:bool)
                        n298 = Equal To 0?(x=w1578) -> (x = 0?=w1577:bool)
                        n299 = Equal To 0?(x=w1579) -> (x = 0?=w1576:bool)
                        n300 = Equal To 0?(x=w1575) -> (x = 0?=w1573:bool)
                        n301 = Equal To 0?(x=w1574) -> (x = 0?=w1572:bool)
                        n302 = Equal To 0?(x=w1570) -> (x = 0?=w1569:bool)
                        n303 = Equal To 0?(x=w1571) -> (x = 0?=w1568:bool)
                        n304 = Equal To 0?(x=w1567) -> (x = 0?=w1565:bool)
                        n305 = Equal To 0?(x=w1566) -> (x = 0?=w1564:bool)
                        n306 = Equal To 0?(x=w1562) -> (x = 0?=w1561:bool)
                        n307 = Equal To 0?(x=w1563) -> (x = 0?=w1560:bool)
                        n308 = Equal To 0?(x=w1559) -> (x = 0?=w1557:bool)
                        n309 = Equal To 0?(x=w1558) -> (x = 0?=w1556:bool)
                        n310 = Equal To 0?(x=w1554) -> (x = 0?=w1553:bool)
                        n311 = Equal To 0?(x=w1555) -> (x = 0?=w1552:bool)
                        n312 = Compound Arithmetic op=OR(w1590, w1589, w1585, w1584, w1581, w1580, w1577, w1576, w1573, w1572, w1569, w1568, w1565, w1564, w1561, w1560, w1557, w1556, w1553, w1552) -> (w1588:bool)
                      }
                    }
                  }
                  frame "rfsputter" {
                    n313 = case shown="10" w1593 {
                      tunnel: [FALSE w1598 w1607 w1620 w1637 w1658 w1683 w1712 w1745 w1782 w1823] -> w1594
                      frame 0, Default {
                      }
                      frame 1 {
                        n314 = local read "rf step length 1"() -> (w1601:dbl)
                        n315 = local read "rf step watt 1"() -> (w1602:dbl)
                        n316 = Equal To 0?(x=w1602) -> (x = 0?=w1600:bool)
                        n317 = Equal To 0?(x=w1601) -> (x = 0?=w1599:bool)
                        n318 = Compound Arithmetic op=OR(w1600, w1599) -> (w1598:bool)
                      }
                      frame 2 {
                        n319 = local read "rf step length 1"() -> (w1610:dbl)
                        n320 = local read "rf step length 2"() -> (w1606:dbl)
                        n321 = local read "rf step watt 1"() -> (w1611:dbl)
                        n322 = local read "rf step watt 2"() -> (w1605:dbl)
                        n323 = Equal To 0?(x=w1611) -> (x = 0?=w1609:bool)
                        n324 = Equal To 0?(x=w1605) -> (x = 0?=w1604:bool)
                        n325 = Equal To 0?(x=w1610) -> (x = 0?=w1608:bool)
                        n326 = Equal To 0?(x=w1606) -> (x = 0?=w1603:bool)
                        n327 = Compound Arithmetic op=OR(w1609, w1608, w1604, w1603) -> (w1607:bool)
                      }
                      frame 3 {
                        n328 = local read "rf step length 1"() -> (w1623:dbl)
                        n329 = local read "rf step length 2"() -> (w1619:dbl)
                        n330 = local read "rf step length 3"() -> (w1614:dbl)
                        n331 = local read "rf step watt 1"() -> (w1624:dbl)
                        n332 = local read "rf step watt 2"() -> (w1618:dbl)
                        n333 = local read "rf step watt 3"() -> (w1615:dbl)
                        n334 = Equal To 0?(x=w1624) -> (x = 0?=w1622:bool)
                        n335 = Equal To 0?(x=w1618) -> (x = 0?=w1617:bool)
                        n336 = Equal To 0?(x=w1623) -> (x = 0?=w1621:bool)
                        n337 = Equal To 0?(x=w1615) -> (x = 0?=w1613:bool)
                        n338 = Equal To 0?(x=w1619) -> (x = 0?=w1616:bool)
                        n339 = Equal To 0?(x=w1614) -> (x = 0?=w1612:bool)
                        n340 = Compound Arithmetic op=OR(w1622, w1621, w1617, w1616, w1613, w1612) -> (w1620:bool)
                      }
                      frame 4 {
                        n341 = local read "rf step length 1"() -> (w1640:dbl)
                        n342 = local read "rf step length 4"() -> (w1628:dbl)
                        n343 = local read "rf step length 2"() -> (w1636:dbl)
                        n344 = local read "rf step length 3"() -> (w1631:dbl)
                        n345 = local read "rf step watt 1"() -> (w1641:dbl)
                        n346 = local read "rf step watt 2"() -> (w1635:dbl)
                        n347 = local read "rf step watt 4"() -> (w1627:dbl)
                        n348 = local read "rf step watt 3"() -> (w1632:dbl)
                        n349 = Equal To 0?(x=w1641) -> (x = 0?=w1639:bool)
                        n350 = Equal To 0?(x=w1635) -> (x = 0?=w1634:bool)
                        n351 = Equal To 0?(x=w1627) -> (x = 0?=w1626:bool)
                        n352 = Equal To 0?(x=w1640) -> (x = 0?=w1638:bool)
                        n353 = Equal To 0?(x=w1632) -> (x = 0?=w1630:bool)
                        n354 = Equal To 0?(x=w1628) -> (x = 0?=w1625:bool)
                        n355 = Equal To 0?(x=w1636) -> (x = 0?=w1633:bool)
                        n356 = Equal To 0?(x=w1631) -> (x = 0?=w1629:bool)
                        n357 = Compound Arithmetic op=OR(w1639, w1638, w1634, w1633, w1630, w1629, w1626, w1625) -> (w1637:bool)
                      }
                      frame 5 {
                        n358 = local read "rf step length 1"() -> (w1661:dbl)
                        n359 = local read "rf step length 2"() -> (w1657:dbl)
                        n360 = local read "rf step length 3"() -> (w1652:dbl)
                        n361 = local read "rf step length 4"() -> (w1649:dbl)
                        n362 = local read "rf step length 5"() -> (w1644:dbl)
                        n363 = local read "rf step watt 1"() -> (w1662:dbl)
                        n364 = local read "rf step watt 2"() -> (w1656:dbl)
                        n365 = local read "rf step watt 3"() -> (w1653:dbl)
                        n366 = local read "rf step watt 4"() -> (w1648:dbl)
                        n367 = local read "rf step watt 5"() -> (w1645:dbl)
                        n368 = Equal To 0?(x=w1662) -> (x = 0?=w1660:bool)
                        n369 = Equal To 0?(x=w1661) -> (x = 0?=w1659:bool)
                        n370 = Equal To 0?(x=w1656) -> (x = 0?=w1655:bool)
                        n371 = Equal To 0?(x=w1657) -> (x = 0?=w1654:bool)
                        n372 = Equal To 0?(x=w1653) -> (x = 0?=w1651:bool)
                        n373 = Equal To 0?(x=w1652) -> (x = 0?=w1650:bool)
                        n374 = Equal To 0?(x=w1648) -> (x = 0?=w1647:bool)
                        n375 = Equal To 0?(x=w1649) -> (x = 0?=w1646:bool)
                        n376 = Equal To 0?(x=w1645) -> (x = 0?=w1643:bool)
                        n377 = Equal To 0?(x=w1644) -> (x = 0?=w1642:bool)
                        n378 = Compound Arithmetic op=OR(w1660, w1659, w1655, w1654, w1651, w1650, w1647, w1646, w1643, w1642) -> (w1658:bool)
                      }
                      frame 6 {
                        n379 = local read "rf step length 3"() -> (w1677:dbl)
                        n380 = local read "rf step length 4"() -> (w1674:dbl)
                        n381 = local read "rf step length 5"() -> (w1669:dbl)
                        n382 = local read "rf step length 6"() -> (w1666:dbl)
                        n383 = local read "rf step length 1"() -> (w1686:dbl)
                        n384 = local read "rf step length 2"() -> (w1682:dbl)
                        n385 = local read "rf step watt 4"() -> (w1673:dbl)
                        n386 = local read "rf step watt 5"() -> (w1670:dbl)
                        n387 = local read "rf step watt 6"() -> (w1665:dbl)
                        n388 = local read "rf step watt 1"() -> (w1687:dbl)
                        n389 = local read "rf step watt 2"() -> (w1681:dbl)
                        n390 = local read "rf step watt 3"() -> (w1678:dbl)
                        n391 = Equal To 0?(x=w1665) -> (x = 0?=w1664:bool)
                        n392 = Equal To 0?(x=w1666) -> (x = 0?=w1663:bool)
                        n393 = Equal To 0?(x=w1670) -> (x = 0?=w1668:bool)
                        n394 = Equal To 0?(x=w1687) -> (x = 0?=w1685:bool)
                        n395 = Equal To 0?(x=w1669) -> (x = 0?=w1667:bool)
                        n396 = Equal To 0?(x=w1681) -> (x = 0?=w1680:bool)
                        n397 = Equal To 0?(x=w1673) -> (x = 0?=w1672:bool)
                        n398 = Equal To 0?(x=w1686) -> (x = 0?=w1684:bool)
                        n399 = Equal To 0?(x=w1678) -> (x = 0?=w1676:bool)
                        n400 = Equal To 0?(x=w1674) -> (x = 0?=w1671:bool)
                        n401 = Equal To 0?(x=w1682) -> (x = 0?=w1679:bool)
                        n402 = Equal To 0?(x=w1677) -> (x = 0?=w1675:bool)
                        n403 = Compound Arithmetic op=OR(w1685, w1684, w1680, w1679, w1676, w1675, w1672, w1671, w1668, w1667, w1664, w1663) -> (w1683:bool)
                      }
                      frame 7 {
                        n404 = local read "rf step length 5"() -> (w1698:dbl)
                        n405 = local read "rf step length 6"() -> (w1695:dbl)
                        n406 = local read "rf step length 7"() -> (w1690:dbl)
                        n407 = local read "rf step length 1"() -> (w1715:dbl)
                        n408 = local read "rf step length 2"() -> (w1711:dbl)
                        n409 = local read "rf step length 3"() -> (w1706:dbl)
                        n410 = local read "rf step length 4"() -> (w1703:dbl)
                        n411 = local read "rf step watt 5"() -> (w1699:dbl)
                        n412 = local read "rf step watt 6"() -> (w1694:dbl)
                        n413 = local read "rf step watt 7"() -> (w1691:dbl)
                        n414 = local read "rf step watt 1"() -> (w1716:dbl)
                        n415 = local read "rf step watt 2"() -> (w1710:dbl)
                        n416 = local read "rf step watt 3"() -> (w1707:dbl)
                        n417 = local read "rf step watt 4"() -> (w1702:dbl)
                        n418 = Equal To 0?(x=w1716) -> (x = 0?=w1714:bool)
                        n419 = Equal To 0?(x=w1715) -> (x = 0?=w1713:bool)
                        n420 = Equal To 0?(x=w1710) -> (x = 0?=w1709:bool)
                        n421 = Equal To 0?(x=w1711) -> (x = 0?=w1708:bool)
                        n422 = Equal To 0?(x=w1707) -> (x = 0?=w1705:bool)
                        n423 = Equal To 0?(x=w1706) -> (x = 0?=w1704:bool)
                        n424 = Equal To 0?(x=w1702) -> (x = 0?=w1701:bool)
                        n425 = Equal To 0?(x=w1703) -> (x = 0?=w1700:bool)
                        n426 = Equal To 0?(x=w1699) -> (x = 0?=w1697:bool)
                        n427 = Equal To 0?(x=w1698) -> (x = 0?=w1696:bool)
                        n428 = Equal To 0?(x=w1694) -> (x = 0?=w1693:bool)
                        n429 = Equal To 0?(x=w1695) -> (x = 0?=w1692:bool)
                        n430 = Equal To 0?(x=w1691) -> (x = 0?=w1689:bool)
                        n431 = Equal To 0?(x=w1690) -> (x = 0?=w1688:bool)
                        n432 = Compound Arithmetic op=OR(w1714, w1713, w1709, w1708, w1705, w1704, w1701, w1700, w1697, w1696, w1693, w1692, w1689, w1688) -> (w1712:bool)
                      }
                      frame 8 {
                        n433 = local read "rf step length 6"() -> (w1728:dbl)
                        n434 = local read "rf step length 7"() -> (w1723:dbl)
                        n435 = local read "rf step length 8"() -> (w1720:dbl)
                        n436 = local read "rf step length 5"() -> (w1731:dbl)
                        n437 = local read "rf step length 1"() -> (w1748:dbl)
                        n438 = local read "rf step length 4"() -> (w1736:dbl)
                        n439 = local read "rf step length 2"() -> (w1744:dbl)
                        n440 = local read "rf step length 3"() -> (w1739:dbl)
                        n441 = local read "rf step watt 6"() -> (w1727:dbl)
                        n442 = local read "rf step watt 7"() -> (w1724:dbl)
                        n443 = local read "rf step watt 8"() -> (w1719:dbl)
                        n444 = local read "rf step watt 5"() -> (w1732:dbl)
                        n445 = local read "rf step watt 1"() -> (w1749:dbl)
                        n446 = local read "rf step watt 2"() -> (w1743:dbl)
                        n447 = local read "rf step watt 4"() -> (w1735:dbl)
                        n448 = local read "rf step watt 3"() -> (w1740:dbl)
                        n449 = Equal To 0?(x=w1727) -> (x = 0?=w1726:bool)
                        n450 = Equal To 0?(x=w1724) -> (x = 0?=w1722:bool)
                        n451 = Equal To 0?(x=w1728) -> (x = 0?=w1725:bool)
                        n452 = Equal To 0?(x=w1723) -> (x = 0?=w1721:bool)
                        n453 = Equal To 0?(x=w1719) -> (x = 0?=w1718:bool)
                        n454 = Equal To 0?(x=w1732) -> (x = 0?=w1730:bool)
                        n455 = Equal To 0?(x=w1720) -> (x = 0?=w1717:bool)
                        n456 = Equal To 0?(x=w1749) -> (x = 0?=w1747:bool)
                        n457 = Equal To 0?(x=w1731) -> (x = 0?=w1729:bool)
                        n458 = Equal To 0?(x=w1743) -> (x = 0?=w1742:bool)
                        n459 = Equal To 0?(x=w1735) -> (x = 0?=w1734:bool)
                        n460 = Equal To 0?(x=w1748) -> (x = 0?=w1746:bool)
                        n461 = Equal To 0?(x=w1740) -> (x = 0?=w1738:bool)
                        n462 = Equal To 0?(x=w1736) -> (x = 0?=w1733:bool)
                        n463 = Equal To 0?(x=w1744) -> (x = 0?=w1741:bool)
                        n464 = Equal To 0?(x=w1739) -> (x = 0?=w1737:bool)
                        n465 = Compound Arithmetic op=OR(w1747, w1746, w1742, w1741, w1738, w1737, w1734, w1733, w1730, w1729, w1726, w1725, w1722, w1721, w1718, w1717) -> (w1745:bool)
                      }
                      frame 9 {
                        n466 = local read "rf step length 1"() -> (w1785:dbl)
                        n467 = local read "rf step length 2"() -> (w1781:dbl)
                        n468 = local read "rf step length 3"() -> (w1776:dbl)
                        n469 = local read "rf step length 4"() -> (w1773:dbl)
                        n470 = local read "rf step length 5"() -> (w1768:dbl)
                        n471 = local read "rf step length 6"() -> (w1765:dbl)
                        n472 = local read "rf step length 7"() -> (w1760:dbl)
                        n473 = local read "rf step length 8"() -> (w1757:dbl)
                        n474 = local read "rf step length 9"() -> (w1752:dbl)
                        n475 = local read "rf step watt 1"() -> (w1786:dbl)
                        n476 = local read "rf step watt 2"() -> (w1780:dbl)
                        n477 = local read "rf step watt 3"() -> (w1777:dbl)
                        n478 = local read "rf step watt 4"() -> (w1772:dbl)
                        n479 = local read "rf step watt 5"() -> (w1769:dbl)
                        n480 = local read "rf step watt 6"() -> (w1764:dbl)
                        n481 = local read "rf step watt 7"() -> (w1761:dbl)
                        n482 = local read "rf step watt 8"() -> (w1756:dbl)
                        n483 = local read "rf step watt 9"() -> (w1753:dbl)
                        n484 = Equal To 0?(x=w1786) -> (x = 0?=w1784:bool)
                        n485 = Equal To 0?(x=w1785) -> (x = 0?=w1783:bool)
                        n486 = Equal To 0?(x=w1780) -> (x = 0?=w1779:bool)
                        n487 = Equal To 0?(x=w1781) -> (x = 0?=w1778:bool)
                        n488 = Equal To 0?(x=w1777) -> (x = 0?=w1775:bool)
                        n489 = Equal To 0?(x=w1776) -> (x = 0?=w1774:bool)
                        n490 = Equal To 0?(x=w1772) -> (x = 0?=w1771:bool)
                        n491 = Equal To 0?(x=w1773) -> (x = 0?=w1770:bool)
                        n492 = Equal To 0?(x=w1769) -> (x = 0?=w1767:bool)
                        n493 = Equal To 0?(x=w1768) -> (x = 0?=w1766:bool)
                        n494 = Equal To 0?(x=w1764) -> (x = 0?=w1763:bool)
                        n495 = Equal To 0?(x=w1765) -> (x = 0?=w1762:bool)
                        n496 = Equal To 0?(x=w1761) -> (x = 0?=w1759:bool)
                        n497 = Equal To 0?(x=w1760) -> (x = 0?=w1758:bool)
                        n498 = Equal To 0?(x=w1756) -> (x = 0?=w1755:bool)
                        n499 = Equal To 0?(x=w1757) -> (x = 0?=w1754:bool)
                        n500 = Equal To 0?(x=w1753) -> (x = 0?=w1751:bool)
                        n501 = Equal To 0?(x=w1752) -> (x = 0?=w1750:bool)
                        n502 = Compound Arithmetic op=OR(w1784, w1783, w1779, w1778, w1775, w1774, w1771, w1770, w1767, w1766, w1763, w1762, w1759, w1758, w1755, w1754, w1751, w1750) -> (w1782:bool)
                      }
                      frame 10 {
                        n503 = local read "rf step length 10"() -> (w1790:dbl)
                        n504 = local read "rf step length 1"() -> (w1826:dbl)
                        n505 = local read "rf step length 2"() -> (w1822:dbl)
                        n506 = local read "rf step length 3"() -> (w1817:dbl)
                        n507 = local read "rf step length 4"() -> (w1814:dbl)
                        n508 = local read "rf step length 5"() -> (w1809:dbl)
                        n509 = local read "rf step length 6"() -> (w1806:dbl)
                        n510 = local read "rf step length 7"() -> (w1801:dbl)
                        n511 = local read "rf step length 8"() -> (w1798:dbl)
                        n512 = local read "rf step length 9"() -> (w1793:dbl)
                        n513 = local read "rf step watt 10"() -> (w1789:dbl)
                        n514 = local read "rf step watt 1"() -> (w1827:dbl)
                        n515 = local read "rf step watt 2"() -> (w1821:dbl)
                        n516 = local read "rf step watt 3"() -> (w1818:dbl)
                        n517 = local read "rf step watt 4"() -> (w1813:dbl)
                        n518 = local read "rf step watt 5"() -> (w1810:dbl)
                        n519 = local read "rf step watt 6"() -> (w1805:dbl)
                        n520 = local read "rf step watt 7"() -> (w1802:dbl)
                        n521 = local read "rf step watt 8"() -> (w1797:dbl)
                        n522 = local read "rf step watt 9"() -> (w1794:dbl)
                        n523 = Equal To 0?(x=w1789) -> (x = 0?=w1788:bool)
                        n524 = Equal To 0?(x=w1790) -> (x = 0?=w1787:bool)
                        n525 = Equal To 0?(x=w1827) -> (x = 0?=w1825:bool)
                        n526 = Equal To 0?(x=w1826) -> (x = 0?=w1824:bool)
                        n527 = Equal To 0?(x=w1821) -> (x = 0?=w1820:bool)
                        n528 = Equal To 0?(x=w1822) -> (x = 0?=w1819:bool)
                        n529 = Equal To 0?(x=w1818) -> (x = 0?=w1816:bool)
                        n530 = Equal To 0?(x=w1817) -> (x = 0?=w1815:bool)
                        n531 = Equal To 0?(x=w1813) -> (x = 0?=w1812:bool)
                        n532 = Equal To 0?(x=w1814) -> (x = 0?=w1811:bool)
                        n533 = Equal To 0?(x=w1810) -> (x = 0?=w1808:bool)
                        n534 = Equal To 0?(x=w1809) -> (x = 0?=w1807:bool)
                        n535 = Equal To 0?(x=w1805) -> (x = 0?=w1804:bool)
                        n536 = Equal To 0?(x=w1806) -> (x = 0?=w1803:bool)
                        n537 = Equal To 0?(x=w1802) -> (x = 0?=w1800:bool)
                        n538 = Equal To 0?(x=w1801) -> (x = 0?=w1799:bool)
                        n539 = Equal To 0?(x=w1797) -> (x = 0?=w1796:bool)
                        n540 = Equal To 0?(x=w1798) -> (x = 0?=w1795:bool)
                        n541 = Equal To 0?(x=w1794) -> (x = 0?=w1792:bool)
                        n542 = Equal To 0?(x=w1793) -> (x = 0?=w1791:bool)
                        n543 = Compound Arithmetic op=OR(w1825, w1824, w1820, w1819, w1816, w1815, w1812, w1811, w1808, w1807, w1804, w1803, w1800, w1799, w1796, w1795, w1792, w1791, w1788, w1787) -> (w1823:bool)
                      }
                    }
                  }
                }
              }
              frame 1 {
                # "multilayer recipe"
              }
            }
            n544 = local read "power rf"() -> (w1320:dbl)
            n545 = Equal To 0?(x=w1320) -> ()  [unwired: 1 out]
            n546 = local read "Pressure set mbar"() -> (w1323:dbl)
            n547 = local read "total length error"() -> (w1325:bool)
            n548 = local read "Ar set sccm"() -> (w1324:dbl)
            n549 = Equal To 0?(x=w1324) -> (x = 0?=w1322:bool)
            n550 = Equal To 0?(x=w1323) -> (x = 0?=w1321:bool)
            n551 = Build Array(FALSE, w1341, w1340, w1338, w1337, w1336, w1335, w1334, w1329, w1328, w1327, w1325, w1322, w1321) -> (w1326:bool[])
            n552 = Boolean Array To Number(Boolean array=w1326) -> (number=w1344:u32)
            n553 = Mantissa & Exponent(0:w1344) -> (2:w1343:dbl)  [unwired: 1 out]
            n554 = case shown="11" w1343 {
              tunnel: [TRUE FALSE FALSE FALSE FALSE FALSE FALSE FALSE FALSE FALSE FALSE FALSE FALSE FALSE] -> w1333
              frame 0, Default {
              }
              frame 1 {
                n555 = One Button Dialog(message="Enter Recipe Name !") -> ()  [unwired: 1 in, 1 out]
              }
              frame 2 {
                n556 = One Button Dialog(message="Enter Substrate Material !") -> ()  [unwired: 1 in, 1 out]
              }
              frame 3 {
                n557 = One Button Dialog(message="Enter Core Diameter !") -> ()  [unwired: 1 in, 1 out]
              }
              frame 4 {
                n558 = One Button Dialog(message="Enter Left Initial Diameter !") -> ()  [unwired: 1 in, 1 out]
              }
              frame 5 {
                n559 = One Button Dialog(message="Enter Web Thickness !") -> ()  [unwired: 1 in, 1 out]
              }
              frame 6 {
                n560 = One Button Dialog(message="Enter Web Speed !") -> ()  [unwired: 1 in, 1 out]
              }
              frame 7 {
                n561 = One Button Dialog(message="Enter Tension Value !") -> ()  [unwired: 1 in, 1 out]
              }
              frame 8 {
                n562 = One Button Dialog(message="Enter Microwave Power !") -> ()  [unwired: 1 in, 1 out]
              }
              frame 9 {
                n563 = One Button Dialog(message="Check DC Step Length(s) and Power(s) !") -> ()  [unwired: 1 in, 1 out]
              }
              frame 10 {
                n564 = One Button Dialog(message="Enter RF Power !") -> ()  [unwired: 1 in, 1 out]
              }
              frame 11 {
                n565 = One Button Dialog(message="Check Step Length(s) !") -> ()  [unwired: 1 in, 1 out]
              }
              frame 12 {
                n566 = One Button Dialog(message="Enter Argon Flow !") -> ()  [unwired: 1 in, 1 out]
              }
              frame 13 {
                n567 = One Button Dialog(message="Enter Pressure  !") -> ()  [unwired: 1 in, 1 out]
              }
            }
            "done" <- w1333
          }
        }
        n568 = case shown="True" "CALCULATE" {
          frame False {
          }
          frame True {
            n569 = stacked-sequence {
              frame #0 {
                n570 = local write "total length"(0.0 ("total length")) -> ()
                "left diameter after roll" <- "left initial diameter"
              }
              frame #1 {
                n571 = while {
                  i -> [w1309]
                  stop <- w1308 stop-if-true
                  n572 = local read "left diameter after roll"() -> (w1307:dbl)
                  n573 = local read "web thickness"() -> (w1305:dbl)
                  n574 = Wait Until Next ms Multiple(millisecond multiple=u32 100) -> ()  [unwired: 1 out]
                  n575 = local read "core diameter"() -> (w1304:dbl)
                  n576 = Multiply(x=w1305, y=0.002) -> (x*y=w1315:dbl)
                  n577 = Multiply(x=3.141592653589793, y=w1307) -> (x*y=w1298:dbl)
                  n578 = Subtract(x=w1307, y=w1315) -> (x-y=w1314:dbl)
                  n579 = local read "CALCULATE"() -> (w1301:bool)
                  n580 = local write "left diameter after roll"(w1314) -> ()
                  n581 = Divide(x=w1298, y=10.0) -> (x/y=w1300:dbl)
                  n582 = Less Or Equal?(x=w1314, y=w1304) -> (x <= y?=w1310:bool)
                  n583 = local read "total length"() -> (w1312:dbl)
                  n584 = Not(x=w1301) -> (.not. x?=w1302:bool)
                  n585 = Greater Or Equal?(x=w1309, y=600) -> (x >= y?=w1306:bool)
                  n586 = Add(x=w1300, y=w1312) -> (x+y=w1313:dbl)
                  n587 = local write "total length"(w1313) -> ()
                  n588 = Compound Arithmetic op=OR(w1310, w1306, w1302) -> (w1308:bool)
                }
              }
              frame #2 {
                n589 = local write "CALCULATE"(FALSE ("CALCULATE")) -> ()
              }
            }
          }
        }
        n590 = local read "single process selection"() -> (w1225:enum32{"microwave", "dcsputter", "rfsputter"})
        n591 = local read "Recipe Selection"() -> (w1237:u16)
        n592 = local read "Web Selection"() -> (w1233:u16)
        n593 = Equal?(x=w1237, y=u16 1) -> (x = y?=w1235:bool)
        n594 = Equal?(x=w1233, y=u16 1) -> (x = y?=w1232:bool)
        n595 = case shown="\"rfsputter\"" w1225 {
          tunnel: [T3."Microwave                " ("single process selection") T3."DC Sputter                   " ("single process selection") T3."RF Sputter                         " ("single process selection")] -> w1224
          tunnel: [FALSE TRUE FALSE] -> w1222
          tunnel: [FALSE FALSE TRUE] -> w1221
          frame "microwave", Default {
          }
          frame "dcsputter" {
          }
          frame "rfsputter" {
          }
        }
        n596 = case shown="True" w1235 {
          tunnel: [T2."Single Recipe                                    " ("recipe selection") T2."Multilayer Recipe                                      " ("recipe selection")] -> w1231
          frame False {
          }
          frame True {
          }
        }
        n597 = case shown="False" w1232 {
          tunnel: [T1."Web                                                    " ("web-other tab") T1."Other                                                      " ("web-other tab")] -> w1230
          frame False {
          }
          frame True {
          }
        }
        n598 = property on="recipe selection" class="TabCtl (strict)"("Value"=w1231) -> ()  [unwired: 2 in, 2 out]
        n599 = property on="web-other tab" class="TabCtl (strict)"("Value"=w1230) -> ()  [unwired: 2 in, 2 out]
        n600 = property on="single process selection" class="TabCtl (strict)"("Value"=w1224) -> ()  [unwired: 2 in, 2 out]
        n601 = property on="steplist tab DC" class="TabCtl (strict)"("Visible"=w1222) -> ()  [unwired: 2 in, 2 out]
        n602 = property on="steplist tab RF" class="TabCtl (strict)"("Visible"=w1221) -> ()  [unwired: 2 in, 2 out]
        n603 = local read "single process selection"() -> (w1220:enum32{"microwave", "dcsputter", "rfsputter"})
        n604 = case shown="\"dcsputter\"" w1220 {
          tunnel: [0.0 w1255 w1279] -> w1229
          frame "microwave", Default {
          }
          frame "rfsputter" {
            n605 = Compound Arithmetic op=ADD("rf step length 1", "rf step length 2", "rf step length 3", "rf step length 4", "rf step length 5", "rf step length 6", "rf step length 7", "rf step length 8", "rf step length 9", "rf step length 10", "rf step length 11", "rf step length 12", "rf step length 13", "rf step length 14", "rf step length 15", "rf step length 16", "rf step length 17", "rf step length 18", "rf step length 19", "rf step length 20") -> (w1255:dbl)
          }
          frame "dcsputter" {
            n606 = Compound Arithmetic op=ADD("dc step length 1", "dc step length 2", "dc step length 3", "dc step length 4", "dc step length 5", "dc step length 6", "dc step length 7", "dc step length 8", "dc step length 9", "dc step length 10", "dc step length 11", "dc step length 12", "dc step length 13", "dc step length 14", "dc step length 15", "dc step length 16", "dc step length 17", "dc step length 18", "dc step length 19", "dc step length 20") -> (w1279:dbl)
          }
        }
        n607 = case shown="True" "CANCEL" {
          tunnel: [FALSE w1240] -> w1217
          frame False {
          }
          frame True {
            n608 = stacked-sequence {
              tunnel: [_ TRUE] -> w1240
              frame #0 {
                n609 = Wait (ms)(milliseconds to wait=u32 500) -> ()  [unwired: 1 out]
              }
              frame #1 {
                w1243 = FALSE ("CALCULATE")
                n610 = local write "CANCEL"(w1243) -> ()
                n611 = local write "CALCULATE"(w1243) -> ()
              }
            }
          }
        }
        n612 = local read "total length"() -> (w1226:dbl)
        n613 = local read "done"() -> (w1219:bool)
        n614 = Greater?(x=w1229, y=w1226) -> ()  [unwired: 1 out]
        n615 = Compound Arithmetic op=OR(w1219, w1217) -> (w1227:bool)
        "total length error" <- FALSE ("total length error")
      }
      n616 = while {
        stop <- w343 stop-if-true
        n617 = local read "done"() -> (w340:bool)
        n618 = Wait Until Next ms Multiple(millisecond multiple=u32 300) -> ()  [unwired: 1 out]
        n619 = case shown="True" w340 {
          tunnel: [FALSE w348] -> w342
          frame False {
          }
          frame True {
            n620 = stacked-sequence {
              seq-local: [w377 _ _ _ _ _ _ _] -> [_ w453 _ _ _ _ _ _]
              seq-local: [_ w451 _ _ _ _ _ _] -> [_ _ w647 _ _ _ _ _]
              seq-local: [_ _ w646 _ _ _ _ _] -> [_ _ _ w759 _ _ _ _]
              seq-local: [_ _ _ w758 _ _ _ _] -> [_ _ _ _ w913 _ _ _]
              seq-local: [_ _ _ _ w912 _ _ _] -> [_ _ _ _ _ w1134 _ _]
              seq-local: [_ _ _ _ _ w1133 _ _] -> [_ _ _ _ _ _ w1199 _]
              tunnel: [_ _ _ _ _ _ _ TRUE] -> w348
              frame #0 {
                w355 = "\t"
                w362 = "\t"
                w369 = "\t"
                w373 = "\t"
                w380 = "\r\n"
                w388 = "\r\n"
                w389 = "\t"
                n621 = local read "Recipe Selection"() -> (w386:u16)
                n622 = local read "Web Selection"() -> (w383:u16)
                n623 = Equal?(x=w386, y=u16 0) -> (x = y?=w385:bool)
                n624 = Equal?(x=w383, y=u16 0) -> (x = y?=w384:bool)
                n625 = local read "core diameter"() -> (w378:dbl)
                n626 = case shown="False" w385 {
                  tunnel: ["Multilayer Recipe" ("string") "Single Recipe" ("string")] -> w359
                  frame False {
                  }
                  frame True {
                  }
                }
                n627 = case shown="False" w384 {
                  tunnel: ["Other" ("string") "Web" ("string")] -> w353
                  frame False {
                  }
                  frame True {
                  }
                }
                n628 = local read "Substrate Material"() -> (w370:string)
                n629 = Number To Decimal String(number=w378) -> (decimal integer string=w349:string)  [unwired: 1 in]
                n630 = local read "Recipe Name"() -> (w391:string)
                n631 = Concatenate Strings(w380, w380) -> (w379:string)
                n632 = Concatenate Strings("Core Diameter(mm)" ("string"), w369, w369, w369, ":" ("string"), "\t", w349, "\r\n") -> (w351:string)
                n633 = Concatenate Strings(w388, w388) -> (w381:string)
                n634 = Concatenate Strings("Recipe Selection" ("string"), w362, w362, w362, ":" ("string"), "\t", w359, "\r\n") -> (w361:string)
                n635 = Concatenate Strings("Recipe Name" ("string"), w389, w389, w389, ":" ("string"), "\t", w391, "\r\n") -> (w392:string)
                n636 = Concatenate Strings("Substrate Material" ("string"), w373, w373, w373, ":" ("string"), "\t", w370, "\r\n") -> (w371:string)
                n637 = Concatenate Strings("Web Selection" ("string"), w355, w355, w355, ":" ("string"), "\t", w353, "\r\n") -> (w352:string)
                n638 = Concatenate Strings(w392, w371, w381, w361, w352, w379, w351) -> (w377:string)
              }
              frame #1 {
                w409 = "\t"
                w416 = "\t"
                w423 = "\t"
                w430 = "\t"
                w437 = "\t"
                w443 = "\t"
                w445 = "\r\n"
                w455 = "\r\n"
                w457 = "\r\n"
                n639 = local read "single process selection"() -> (w447:enum32{"microwave", "dcsputter", "rfsputter"})
                n640 = local read "web thickness"() -> (w450:dbl)
                n641 = local read "left initial diameter"() -> (w401:dbl)
                n642 = case shown="\"dcsputter\"" w447 {
                  tunnel: ["Microwave" ("string") "DC Sputter" ("string") "RF Sputter" ("string")] -> w410
                  tunnel: [FALSE TRUE FALSE] -> w446
                  frame "microwave", Default {
                  }
                  frame "dcsputter" {
                  }
                  frame "rfsputter" {
                  }
                }
                n643 = local read "web speed"() -> (w449:dbl)
                n644 = local read "tension value"() -> (w448:dbl)
                n645 = Number To Decimal String(number=w450) -> (decimal integer string=w433:string)  [unwired: 1 in]
                n646 = Format Into String(format string="%.;%f", w401) -> (resulting string=w400:string)  [unwired: 2 in, 1 out]
                n647 = Number To Decimal String(number=w449) -> (decimal integer string=w424:string)  [unwired: 1 in]
                n648 = Number To Decimal String(number=w448) -> (decimal integer string=w417:string)  [unwired: 1 in]
                n649 = Concatenate Strings(w455, w455) -> (w454:string)
                n650 = Concatenate Strings("Web Thickness(µm)" ("string"), w437, w437, w437, ":" ("string"), "\t", w433, "\r\n") -> (w432:string)
                n651 = case shown="True" w446 {
                  tunnel: ["NULL" ("string") w459] -> w403
                  frame False {
                  }
                  frame True {
                    n652 = local read "DC Sputter Chamber Selection"() -> (w460:enum32{"chamber II", "chamber III"})
                    n653 = case shown="\"chamber II\", Default" w460 {
                      tunnel: ["II" ("string") "III" ("string")] -> w459
                      frame "chamber II", Default {
                      }
                      frame "chamber III" {
                      }
                    }
                  }
                }
                n654 = Concatenate Strings(w457, w457) -> (w456:string)
                n655 = Concatenate Strings("Web Speed(cm/min)" ("string"), w430, w430, w430, ":" ("string"), "\t", w424, "\r\n") -> (w426:string)
                n656 = Concatenate Strings("Tension Value(N)" ("string"), w423, w423, w423, ":" ("string"), "\t", w417, "\r\n") -> (w419:string)
                n657 = Concatenate Strings("Left Initial Diameter(mm)" ("string"), w443, w443, w443, ":" ("string"), "\t", w400, "\r\n") -> (w439:string)
                n658 = Concatenate Strings("Single Process Selection" ("string"), w416, w416, w416, ":" ("string"), "\t", w410, "\r\n") -> (w412:string)
                n659 = Concatenate Strings(w445, w445) -> (w444:string)
                n660 = Concatenate Strings("Chamber Selection" ("string"), w409, w409, w409, ":" ("string"), "\t", w403, "\r\n") -> (w405:string)
                n661 = Concatenate Strings(w439, w432, w456, w426, w419, w454, w412, w405, w444) -> (w452:string)
                n662 = Concatenate Strings(w453, w452) -> (w451:string)
              }
              frame #2 {
                w520 = "\t"
                w515 = "\t"
                w510 = "\t"
                w505 = "\t"
                w500 = "\t"
                w495 = "\t"
                w490 = "\t"
                w485 = "\t"
                w480 = "\t"
                w475 = "\t"
                w560 = "\t"
                w552 = "\t"
                w605 = "\t"
                w619 = "\t"
                w624 = "\t"
                w616 = "\t"
                w611 = "\t"
                w632 = "\t"
                w627 = "\t"
                w635 = "\t"
                w640 = "\t"
                w643 = "\r\n"
                w645 = "\r\n"
                w651 = "\r\n"
                n663 = local read "dc step watt 4"() -> (w630:dbl)
                n664 = local read "dc step watt 1"() -> (w638:dbl)
                n665 = local read "dc step watt 2"() -> (w637:dbl)
                n666 = local read "dc step watt 3"() -> (w629:dbl)
                n667 = local read "dc step watt 5"() -> (w607:dbl)
                n668 = local read "dc step watt 14"() -> (w549:dbl)
                n669 = local read "dc step watt 12"() -> (w550:dbl)
                n670 = local read "dc step watt 13"() -> (w548:dbl)
                n671 = local read "dc step watt 11"() -> (w551:dbl)
                n672 = local read "dc step watt 15"() -> (w542:dbl)
                n673 = Number To Decimal String(number=w630) -> (decimal integer string=w574:string)  [unwired: 1 in]
                n674 = Number To Decimal String(number=w637) -> (decimal integer string=w578:string)  [unwired: 1 in]
                n675 = Number To Decimal String(number=w629) -> (decimal integer string=w576:string)  [unwired: 1 in]
                n676 = Number To Decimal String(number=w638) -> (decimal integer string=w580:string)  [unwired: 1 in]
                n677 = Number To Decimal String(number=w607) -> (decimal integer string=w572:string)  [unwired: 1 in]
                n678 = Number To Decimal String(number=w549) -> (decimal integer string=w528:string)  [unwired: 1 in]
                n679 = Number To Decimal String(number=w550) -> (decimal integer string=w530:string)  [unwired: 1 in]
                n680 = Number To Decimal String(number=w548) -> (decimal integer string=w529:string)  [unwired: 1 in]
                n681 = Number To Decimal String(number=w551) -> (decimal integer string=w531:string)  [unwired: 1 in]
                n682 = Number To Decimal String(number=w542) -> (decimal integer string=w527:string)  [unwired: 1 in]
                n683 = local read "power microwave"() -> (w649:dbl)
                n684 = Number To Decimal String(number=w649) -> (decimal integer string=w555:string)  [unwired: 1 in]
                n685 = Concatenate Strings("DC Step 4 power" ("string"), w632, w632, w632, ":" ("string"), "\t", w574, "\r\n") -> (w600:string)
                n686 = Concatenate Strings("DC Step 5 power" ("string"), w605, w605, w605, ":" ("string"), "\t", w572, "\r\n") -> (w599:string)
                n687 = Concatenate Strings("DC Step 2 power" ("string"), w635, w635, w635, ":" ("string"), "\t", w578, "\r\n") -> (w602:string)
                n688 = Concatenate Strings("DC Step 3 power" ("string"), w627, w627, w627, ":" ("string"), "\t", w576, "\r\n") -> (w601:string)
                n689 = Concatenate Strings("DC Step 1 power" ("string"), w640, w640, w640, ":" ("string"), "\t", w580, "\r\n") -> (w603:string)
                n690 = Concatenate Strings("DC Step 14 power" ("string"), w490, w490, w490, ":" ("string"), "\t", w528, "\r\n") -> (w538:string)
                n691 = Concatenate Strings("DC Step 15 power" ("string"), w515, w515, w515, ":" ("string"), "\t", w527, "\r\n") -> (w537:string)
                n692 = Concatenate Strings("DC Step 12 power" ("string"), w480, w480, w480, ":" ("string"), "\t", w530, "\r\n") -> (w540:string)
                n693 = Concatenate Strings("DC Step 13 power" ("string"), w485, w485, w485, ":" ("string"), "\t", w529, "\r\n") -> (w539:string)
                n694 = Concatenate Strings("DC Step 11 power" ("string"), w475, w475, w475, ":" ("string"), "\t", w531, "\r\n") -> (w541:string)
                n695 = Concatenate Strings("DC Power Steps(power-length)" ("string"), w643, w643) -> (w642:string)
                n696 = Concatenate Strings(w603, w602, w601, w600, w599) -> (w592:string)
                n697 = Concatenate Strings(w651, w651) -> (w650:string)
                n698 = Concatenate Strings(w541, w540, w539, w538, w537) -> (w470:string)
                n699 = Concatenate Strings(w645, w645) -> (w561:string)
                n700 = Concatenate Strings("Microwave Power(watt)" ("string"), w560, w560, w560, ":" ("string"), "\t", w555, "\r\n") -> (w556:string)
                n701 = local read "dc step watt 10"() -> (w608:dbl)
                n702 = local read "dc step watt 9"() -> (w621:dbl)
                n703 = local read "dc step watt 7"() -> (w614:dbl)
                n704 = local read "dc step watt 8"() -> (w622:dbl)
                n705 = local read "dc step watt 6"() -> (w613:dbl)
                n706 = local read "dc step watt 19"() -> (w546:dbl)
                n707 = local read "dc step watt 20"() -> (w543:dbl)
                n708 = local read "dc step watt 17"() -> (w545:dbl)
                n709 = local read "dc step watt 18"() -> (w547:dbl)
                n710 = local read "dc step watt 16"() -> (w544:dbl)
                n711 = Number To Decimal String(number=w621) -> (decimal integer string=w568:string)  [unwired: 1 in]
                n712 = Number To Decimal String(number=w608) -> (decimal integer string=w570:string)  [unwired: 1 in]
                n713 = Number To Decimal String(number=w614) -> (decimal integer string=w564:string)  [unwired: 1 in]
                n714 = Number To Decimal String(number=w622) -> (decimal integer string=w566:string)  [unwired: 1 in]
                n715 = Number To Decimal String(number=w613) -> (decimal integer string=w562:string)  [unwired: 1 in]
                n716 = Number To Decimal String(number=w546) -> (decimal integer string=w525:string)  [unwired: 1 in]
                n717 = Number To Decimal String(number=w543) -> (decimal integer string=w526:string)  [unwired: 1 in]
                n718 = Number To Decimal String(number=w545) -> (decimal integer string=w523:string)  [unwired: 1 in]
                n719 = Number To Decimal String(number=w547) -> (decimal integer string=w524:string)  [unwired: 1 in]
                n720 = Number To Decimal String(number=w544) -> (decimal integer string=w522:string)  [unwired: 1 in]
                n721 = Concatenate Strings("DC Step 9 power" ("string"), w619, w619, w619, ":" ("string"), "\t", w568, "\r\n") -> (w595:string)
                n722 = Concatenate Strings("DC Step 10 power" ("string"), w552, w552, w552, ":" ("string"), "\t", w570, "\r\n") -> (w594:string)
                n723 = Concatenate Strings("DC Step 7 power" ("string"), w616, w616, w616, ":" ("string"), "\t", w564, "\r\n") -> (w597:string)
                n724 = Concatenate Strings("DC Step 8 power" ("string"), w624, w624, w624, ":" ("string"), "\t", w566, "\r\n") -> (w596:string)
                n725 = Concatenate Strings("DC Step 6 power" ("string"), w611, w611, w611, ":" ("string"), "\t", w562, "\r\n") -> (w598:string)
                n726 = Concatenate Strings("DC Step 19 power" ("string"), w510, w510, w510, ":" ("string"), "\t", w525, "\r\n") -> (w533:string)
                n727 = Concatenate Strings("DC Step 20 power" ("string"), w520, w520, w520, ":" ("string"), "\t", w526, "\r\n") -> (w532:string)
                n728 = Concatenate Strings("DC Step 17 power" ("string"), w500, w500, w500, ":" ("string"), "\t", w523, "\r\n") -> (w535:string)
                n729 = Concatenate Strings("DC Step 18 power" ("string"), w505, w505, w505, ":" ("string"), "\t", w524, "\r\n") -> (w534:string)
                n730 = Concatenate Strings("DC Step 16 power" ("string"), w495, w495, w495, ":" ("string"), "\t", w522, "\r\n") -> (w536:string)
                n731 = Concatenate Strings(w536, w535, w534, w533, w532) -> (w471:string)
                n732 = Concatenate Strings(w470, w471) -> (w469:string)
                n733 = Concatenate Strings(w598, w597, w596, w595, w594, w469) -> (w593:string)
                n734 = Concatenate Strings(w556, w561, w650, w642, w592, w593) -> (w648:string)
                n735 = Concatenate Strings(w647, w648) -> (w646:string)
              }
              frame #3 {
                w694 = "\t"
                w691 = "\t"
                w689 = "\t"
                w687 = "\t"
                w656 = "\t"
                w733 = "\t"
                w731 = "\t"
                w729 = "\t"
                w726 = "\t"
                w727 = "\t"
                w756 = "\r\n"
                w736 = "\t"
                w747 = "\t"
                w739 = "\t"
                w741 = "\t"
                w743 = "\t"
                w744 = "\t"
                w749 = "\t"
                w751 = "\t"
                w754 = "\t"
                w753 = "\t"
                n736 = local read "dc step length 4"() -> (w814:dbl)
                n737 = local read "dc step length 2"() -> (w817:dbl)
                n738 = local read "dc step length 3"() -> (w813:dbl)
                n739 = local read "dc step length 1"() -> (w818:dbl)
                n740 = local read "dc step length 5"() -> (w801:dbl)
                n741 = local read "dc step length 14"() -> (w700:dbl)
                n742 = local read "dc step length 12"() -> (w697:dbl)
                n743 = local read "dc step length 13"() -> (w701:dbl)
                n744 = local read "dc step length 11"() -> (w696:dbl)
                n745 = local read "dc step length 15"() -> (w703:dbl)
                n746 = Number To Decimal String(number=w814) -> (decimal integer string=w772:string)  [unwired: 1 in]
                n747 = Number To Decimal String(number=w817) -> (decimal integer string=w776:string)  [unwired: 1 in]
                n748 = Number To Decimal String(number=w813) -> (decimal integer string=w774:string)  [unwired: 1 in]
                n749 = Number To Decimal String(number=w818) -> (decimal integer string=w778:string)  [unwired: 1 in]
                n750 = Number To Decimal String(number=w801) -> (decimal integer string=w770:string)  [unwired: 1 in]
                n751 = Number To Decimal String(number=w700) -> (decimal integer string=w722:string)  [unwired: 1 in]
                n752 = Number To Decimal String(number=w697) -> (decimal integer string=w718:string)  [unwired: 1 in]
                n753 = Number To Decimal String(number=w701) -> (decimal integer string=w720:string)  [unwired: 1 in]
                n754 = Number To Decimal String(number=w696) -> (decimal integer string=w716:string)  [unwired: 1 in]
                n755 = Number To Decimal String(number=w703) -> (decimal integer string=w724:string)  [unwired: 1 in]
                n756 = Concatenate Strings("DC Step 4 length" ("string"), w749, w749, w749, ":" ("string"), "\t", w772, "\r\n") -> (w796:string)
                n757 = Concatenate Strings("DC Step 5 length" ("string"), w747, w747, w747, ":" ("string"), "\t", w770, "\r\n") -> (w795:string)
                n758 = Concatenate Strings("DC Step 2 length" ("string"), w754, w754, w754, ":" ("string"), "\t", w776, "\r\n") -> (w798:string)
                n759 = Concatenate Strings("DC Step 3 length" ("string"), w751, w751, w751, ":" ("string"), "\t", w774, "\r\n") -> (w797:string)
                n760 = Concatenate Strings("DC Step 1 length" ("string"), w753, w753, w753, ":" ("string"), "\t", w778, "\r\n") -> (w799:string)
                n761 = Concatenate Strings("DC Step 14 length" ("string"), w731, w731, w731, ":" ("string"), "\t", w722, "\r\n") -> (w708:string)
                n762 = Concatenate Strings("DC Step 15 length" ("string"), w733, w733, w733, ":" ("string"), "\t", w724, "\r\n") -> (w709:string)
                n763 = Concatenate Strings("DC Step 12 length" ("string"), w726, w726, w726, ":" ("string"), "\t", w718, "\r\n") -> (w706:string)
                n764 = Concatenate Strings("DC Step 13 length" ("string"), w729, w729, w729, ":" ("string"), "\t", w720, "\r\n") -> (w707:string)
                n765 = Concatenate Strings("DC Step 11 length" ("string"), w727, w727, w727, ":" ("string"), "\t", w716, "\r\n") -> (w705:string)
                n766 = Concatenate Strings(w799, w798, w797, w796, w795) -> (w757:string)
                n767 = Concatenate Strings(w705, w706, w707, w708, w709) -> (w654:string)
                n768 = local read "dc step length 10"() -> (w802:dbl)
                n769 = local read "dc step length 9"() -> (w809:dbl)
                n770 = local read "dc step length 7"() -> (w806:dbl)
                n771 = local read "dc step length 8"() -> (w810:dbl)
                n772 = local read "dc step length 6"() -> (w805:dbl)
                n773 = local read "dc step length 19"() -> (w659:dbl)
                n774 = local read "dc step length 20"() -> (w666:dbl)
                n775 = local read "dc step length 17"() -> (w662:dbl)
                n776 = local read "dc step length 18"() -> (w658:dbl)
                n777 = local read "dc step length 16"() -> (w663:dbl)
                n778 = Number To Decimal String(number=w809) -> (decimal integer string=w766:string)  [unwired: 1 in]
                n779 = Number To Decimal String(number=w802) -> (decimal integer string=w768:string)  [unwired: 1 in]
                n780 = Number To Decimal String(number=w806) -> (decimal integer string=w762:string)  [unwired: 1 in]
                n781 = Number To Decimal String(number=w810) -> (decimal integer string=w764:string)  [unwired: 1 in]
                n782 = Number To Decimal String(number=w805) -> (decimal integer string=w760:string)  [unwired: 1 in]
                n783 = Number To Decimal String(number=w659) -> (decimal integer string=w680:string)  [unwired: 1 in]
                n784 = Number To Decimal String(number=w666) -> (decimal integer string=w678:string)  [unwired: 1 in]
                n785 = Number To Decimal String(number=w662) -> (decimal integer string=w684:string)  [unwired: 1 in]
                n786 = Number To Decimal String(number=w658) -> (decimal integer string=w682:string)  [unwired: 1 in]
                n787 = Number To Decimal String(number=w663) -> (decimal integer string=w686:string)  [unwired: 1 in]
                n788 = Concatenate Strings("DC Step 9 length" ("string"), w739, w739, w739, ":" ("string"), "\t", w766, "\r\n") -> (w791:string)
                n789 = Concatenate Strings("DC Step 10 length" ("string"), w736, w736, w736, ":" ("string"), "\t", w768, "\r\n") -> (w790:string)
                n790 = Concatenate Strings("DC Step 7 length" ("string"), w743, w743, w743, ":" ("string"), "\t", w762, "\r\n") -> (w793:string)
                n791 = Concatenate Strings("DC Step 8 length" ("string"), w741, w741, w741, ":" ("string"), "\t", w764, "\r\n") -> (w792:string)
                n792 = Concatenate Strings("DC Step 6 length" ("string"), w744, w744, w744, ":" ("string"), "\t", w760, "\r\n") -> (w794:string)
                n793 = Concatenate Strings("DC Step 19 length" ("string"), w691, w691, w691, ":" ("string"), "\t", w680, "\r\n") -> (w670:string)
                n794 = Concatenate Strings("DC Step 20 length" ("string"), w694, w694, w694, ":" ("string"), "\t", w678, "\r\n") -> (w671:string)
                n795 = Concatenate Strings("DC Step 17 length" ("string"), w687, w687, w687, ":" ("string"), "\t", w684, "\r\n") -> (w668:string)
                n796 = Concatenate Strings("DC Step 18 length" ("string"), w689, w689, w689, ":" ("string"), "\t", w682, "\r\n") -> (w669:string)
                n797 = Concatenate Strings("DC Step 16 length" ("string"), w656, w656, w656, ":" ("string"), "\t", w686, "\r\n") -> (w667:string)
                n798 = Concatenate Strings(w794, w793, w792, w791, w790) -> (w735:string)
                n799 = Concatenate Strings(w667, w668, w669, w670, w671) -> (w653:string)
                n800 = Concatenate Strings(w654, w653) -> (w652:string)
                n801 = Concatenate Strings(w756, w756, w757, w735, w652) -> (w820:string)
                n802 = Concatenate Strings(w759, w820) -> (w758:string)
              }
              frame #4 {
                w901 = "\t"
                w857 = "\t"
                w862 = "\t"
                w867 = "\t"
                w872 = "\t"
                w877 = "\t"
                w882 = "\t"
                w887 = "\t"
                w892 = "\t"
                w897 = "\t"
                w908 = "\r\n"
                w910 = "\r\n"
                w904 = "\t"
                w957 = "\t"
                w952 = "\t"
                w947 = "\t"
                w942 = "\t"
                w937 = "\t"
                w932 = "\t"
                w927 = "\t"
                w922 = "\t"
                w917 = "\t"
                n803 = local read "rf step watt 10"() -> (w983:dbl)
                n804 = local read "rf step watt 9"() -> (w986:dbl)
                n805 = local read "rf step watt 7"() -> (w985:dbl)
                n806 = local read "rf step watt 8"() -> (w987:dbl)
                n807 = local read "rf step watt 6"() -> (w984:dbl)
                n808 = local read "rf step watt 4"() -> (w989:dbl)
                n809 = local read "rf step watt 2"() -> (w990:dbl)
                n810 = local read "rf step watt 3"() -> (w988:dbl)
                n811 = local read "rf step watt 1"() -> (w991:dbl)
                n812 = local read "rf step watt 5"() -> (w982:dbl)
                n813 = Number To Decimal String(number=w986) -> (decimal integer string=w965:string)  [unwired: 1 in]
                n814 = Number To Decimal String(number=w983) -> (decimal integer string=w966:string)  [unwired: 1 in]
                n815 = Number To Decimal String(number=w985) -> (decimal integer string=w963:string)  [unwired: 1 in]
                n816 = Number To Decimal String(number=w987) -> (decimal integer string=w964:string)  [unwired: 1 in]
                n817 = Number To Decimal String(number=w984) -> (decimal integer string=w962:string)  [unwired: 1 in]
                n818 = Number To Decimal String(number=w989) -> (decimal integer string=w968:string)  [unwired: 1 in]
                n819 = Number To Decimal String(number=w990) -> (decimal integer string=w970:string)  [unwired: 1 in]
                n820 = Number To Decimal String(number=w988) -> (decimal integer string=w969:string)  [unwired: 1 in]
                n821 = Number To Decimal String(number=w991) -> (decimal integer string=w971:string)  [unwired: 1 in]
                n822 = Number To Decimal String(number=w982) -> (decimal integer string=w967:string)  [unwired: 1 in]
                n823 = Concatenate Strings("RF Step 9 power" ("string"), w952, w952, w952, ":" ("string"), "\t", w965, "\r\n") -> (w973:string)
                n824 = Concatenate Strings("RF Step 10 power" ("string"), w904, w904, w904, ":" ("string"), "\t", w966, "\r\n") -> (w972:string)
                n825 = Concatenate Strings("RF Step 7 power" ("string"), w942, w942, w942, ":" ("string"), "\t", w963, "\r\n") -> (w975:string)
                n826 = Concatenate Strings("RF Step 8 power" ("string"), w947, w947, w947, ":" ("string"), "\t", w964, "\r\n") -> (w974:string)
                n827 = Concatenate Strings("RF Step 6 power" ("string"), w937, w937, w937, ":" ("string"), "\t", w962, "\r\n") -> (w976:string)
                n828 = Concatenate Strings("RF Step 4 power" ("string"), w932, w932, w932, ":" ("string"), "\t", w968, "\r\n") -> (w978:string)
                n829 = Concatenate Strings("RF Step 5 power" ("string"), w957, w957, w957, ":" ("string"), "\t", w967, "\r\n") -> (w977:string)
                n830 = Concatenate Strings("RF Step 2 power" ("string"), w922, w922, w922, ":" ("string"), "\t", w970, "\r\n") -> (w980:string)
                n831 = Concatenate Strings("RF Step 3 power" ("string"), w927, w927, w927, ":" ("string"), "\t", w969, "\r\n") -> (w979:string)
                n832 = Concatenate Strings("RF Step 1 power" ("string"), w917, w917, w917, ":" ("string"), "\t", w971, "\r\n") -> (w981:string)
                n833 = Concatenate Strings("RF Power Steps(power-length)" ("string"), w908, w908) -> (w907:string)
                n834 = Concatenate Strings(w981, w980, w979, w978, w977) -> (w906:string)
                n835 = Concatenate Strings(w976, w975, w974, w973, w972) -> (w905:string)
                n836 = local read "rf step watt 19"() -> (w828:dbl)
                n837 = local read "rf step watt 20"() -> (w831:dbl)
                n838 = local read "rf step watt 17"() -> (w829:dbl)
                n839 = local read "rf step watt 18"() -> (w827:dbl)
                n840 = local read "rf step watt 16"() -> (w830:dbl)
                n841 = local read "rf step watt 14"() -> (w825:dbl)
                n842 = local read "rf step watt 12"() -> (w824:dbl)
                n843 = local read "rf step watt 13"() -> (w826:dbl)
                n844 = local read "rf step watt 11"() -> (w823:dbl)
                n845 = local read "rf step watt 15"() -> (w832:dbl)
                n846 = Number To Decimal String(number=w828) -> (decimal integer string=w849:string)  [unwired: 1 in]
                n847 = Number To Decimal String(number=w831) -> (decimal integer string=w848:string)  [unwired: 1 in]
                n848 = Number To Decimal String(number=w829) -> (decimal integer string=w851:string)  [unwired: 1 in]
                n849 = Number To Decimal String(number=w827) -> (decimal integer string=w850:string)  [unwired: 1 in]
                n850 = Number To Decimal String(number=w830) -> (decimal integer string=w852:string)  [unwired: 1 in]
                n851 = Number To Decimal String(number=w825) -> (decimal integer string=w846:string)  [unwired: 1 in]
                n852 = Number To Decimal String(number=w824) -> (decimal integer string=w844:string)  [unwired: 1 in]
                n853 = Number To Decimal String(number=w826) -> (decimal integer string=w845:string)  [unwired: 1 in]
                n854 = Number To Decimal String(number=w823) -> (decimal integer string=w843:string)  [unwired: 1 in]
                n855 = Number To Decimal String(number=w832) -> (decimal integer string=w847:string)  [unwired: 1 in]
                n856 = Concatenate Strings("RF Step 19 power" ("string"), w862, w862, w862, ":" ("string"), "\t", w849, "\r\n") -> (w841:string)
                n857 = Concatenate Strings("RF Step 20 power" ("string"), w901, w901, w901, ":" ("string"), "\t", w848, "\r\n") -> (w842:string)
                n858 = Concatenate Strings("RF Step 17 power" ("string"), w872, w872, w872, ":" ("string"), "\t", w851, "\r\n") -> (w839:string)
                n859 = Concatenate Strings("RF Step 18 power" ("string"), w867, w867, w867, ":" ("string"), "\t", w850, "\r\n") -> (w840:string)
                n860 = Concatenate Strings("RF Step 16 power" ("string"), w877, w877, w877, ":" ("string"), "\t", w852, "\r\n") -> (w838:string)
                n861 = Concatenate Strings("RF Step 14 power" ("string"), w882, w882, w882, ":" ("string"), "\t", w846, "\r\n") -> (w836:string)
                n862 = Concatenate Strings("RF Step 15 power" ("string"), w857, w857, w857, ":" ("string"), "\t", w847, "\r\n") -> (w837:string)
                n863 = Concatenate Strings("RF Step 12 power" ("string"), w892, w892, w892, ":" ("string"), "\t", w844, "\r\n") -> (w834:string)
                n864 = Concatenate Strings("RF Step 13 power" ("string"), w887, w887, w887, ":" ("string"), "\t", w845, "\r\n") -> (w835:string)
                n865 = Concatenate Strings("RF Step 11 power" ("string"), w897, w897, w897, ":" ("string"), "\t", w843, "\r\n") -> (w833:string)
                n866 = Concatenate Strings(w833, w834, w835, w836, w837) -> (w822:string)
                n867 = Concatenate Strings(w838, w839, w840, w841, w842) -> (w821:string)
                n868 = Concatenate Strings(w910, w910, w907, w906, w905, w822, w821) -> (w911:string)
                n869 = Concatenate Strings(w913, w911) -> (w912:string)
              }
              frame #5 {
                w1056 = "\t"
                w1066 = "\t"
                w1059 = "\t"
                w1061 = "\t"
                w1062 = "\t"
                w1064 = "\t"
                w1069 = "\t"
                w1071 = "\t"
                w1073 = "\t"
                w1074 = "\t"
                w1081 = "\t"
                w1088 = "\r\n"
                w1092 = "\t"
                w1098 = "\r\n"
                w1101 = "\t"
                w1110 = "\t"
                w1135 = "\r\n"
                w1131 = "\t"
                w1121 = "\t"
                w1128 = "\t"
                w1126 = "\t"
                w1125 = "\t"
                w1123 = "\t"
                w1118 = "\t"
                w1116 = "\t"
                w1114 = "\t"
                w1113 = "\t"
                n870 = local read "rf step length 10"() -> (w1179:dbl)
                n871 = local read "rf step length 9"() -> (w1186:dbl)
                n872 = local read "rf step length 7"() -> (w1183:dbl)
                n873 = local read "Pressure set mbar"() -> (w1095:dbl)
                n874 = local read "rf step length 8"() -> (w1187:dbl)
                n875 = local read "rf step length 6"() -> (w1182:dbl)
                n876 = local read "Step Number DC"() -> (w1079:u16)
                n877 = local read "rf step length 4"() -> (w1191:dbl)
                n878 = local read "rf step length 2"() -> (w1194:dbl)
                n879 = local read "rf step length 3"() -> (w1190:dbl)
                n880 = local read "rf step length 1"() -> (w1195:dbl)
                n881 = local read "rf step length 5"() -> (w1178:dbl)
                n882 = local read "Step Number RF"() -> (w1086:u16)
                n883 = local read "Ar set sccm"() -> (w1105:dbl)
                n884 = Number To Decimal String(number=w1186) -> (decimal integer string=w1143:string)  [unwired: 1 in]
                n885 = Number To Decimal String(number=w1179) -> (decimal integer string=w1145:string)  [unwired: 1 in]
                n886 = Number To Decimal String(number=w1183) -> (decimal integer string=w1139:string)  [unwired: 1 in]
                n887 = Number To Decimal String(number=w1187) -> (decimal integer string=w1141:string)  [unwired: 1 in]
                n888 = Number To Decimal String(number=w1182) -> (decimal integer string=w1137:string)  [unwired: 1 in]
                n889 = Number To Decimal String(number=w1191) -> (decimal integer string=w1149:string)  [unwired: 1 in]
                n890 = Number To Decimal String(number=w1194) -> (decimal integer string=w1153:string)  [unwired: 1 in]
                n891 = Number To Decimal String(number=w1190) -> (decimal integer string=w1151:string)  [unwired: 1 in]
                n892 = Number To Decimal String(number=w1195) -> (decimal integer string=w1155:string)  [unwired: 1 in]
                n893 = Number To Decimal String(number=w1079) -> (decimal integer string=w1078:string)  [unwired: 1 in]
                n894 = Number To Decimal String(number=w1178) -> (decimal integer string=w1147:string)  [unwired: 1 in]
                n895 = Number To Decimal String(number=w1105) -> (decimal integer string=w1109:string)  [unwired: 1 in]
                n896 = Format Into String(format string="%.;%f", w1095) -> (resulting string=w1094:string)  [unwired: 2 in, 1 out]
                n897 = Number To Decimal String(number=w1086) -> (decimal integer string=w1085:string)  [unwired: 1 in]
                n898 = Concatenate Strings("RF Step 9 length" ("string"), w1128, w1128, w1128, ":" ("string"), "\t", w1143, "\r\n") -> (w1168:string)
                n899 = Concatenate Strings("RF Step 10 length" ("string"), w1131, w1131, w1131, ":" ("string"), "\t", w1145, "\r\n") -> (w1167:string)
                n900 = Concatenate Strings("RF Step 7 length" ("string"), w1125, w1125, w1125, ":" ("string"), "\t", w1139, "\r\n") -> (w1170:string)
                n901 = Concatenate Strings("RF Step 8 length" ("string"), w1126, w1126, w1126, ":" ("string"), "\t", w1141, "\r\n") -> (w1169:string)
                n902 = Concatenate Strings("RF Step 6 length" ("string"), w1123, w1123, w1123, ":" ("string"), "\t", w1137, "\r\n") -> (w1171:string)
                n903 = Concatenate Strings("RF Step 4 length" ("string"), w1118, w1118, w1118, ":" ("string"), "\t", w1149, "\r\n") -> (w1173:string)
                n904 = Concatenate Strings("RF Step 5 length" ("string"), w1121, w1121, w1121, ":" ("string"), "\t", w1147, "\r\n") -> (w1172:string)
                n905 = Concatenate Strings("RF Step 2 length" ("string"), w1114, w1114, w1114, ":" ("string"), "\t", w1153, "\r\n") -> (w1175:string)
                n906 = Concatenate Strings("RF Step 3 length" ("string"), w1116, w1116, w1116, ":" ("string"), "\t", w1151, "\r\n") -> (w1174:string)
                n907 = Concatenate Strings("RF Step 1 length" ("string"), w1113, w1113, w1113, ":" ("string"), "\t", w1155, "\r\n") -> (w1176:string)
                n908 = Concatenate Strings("Argon Flow(sccm)" ("string"), w1110, w1110, w1110, ":" ("string"), "\t", w1109, "\r\n") -> (w1099:string)
                n909 = Concatenate Strings("Pressure(mbarr)" ("string"), w1101, w1101, w1101, ":" ("string"), "\t", w1094, "\r\n") -> (w1097:string)
                n910 = Concatenate Strings("RF Step Number " ("string"), w1092, w1092, w1092, ":" ("string"), "\t", w1085, "\r\n") -> (w1087:string)
                n911 = Concatenate Strings("DC Step Number" ("string"), w1081, w1081, w1081, ":" ("string"), "\t", w1078, "\r\n") -> (w1077:string)
                n912 = Concatenate Strings(w1176, w1175, w1174, w1173, w1172) -> (w1136:string)
                n913 = Concatenate Strings(w1171, w1170, w1169, w1168, w1167) -> (w1132:string)
                n914 = Concatenate Strings(w1088, w1088, w1087, w1077) -> (w1076:string)
                n915 = Concatenate Strings(w1098, w1098, w1099, w1097, w1076) -> (w992:string)
                n916 = local read "rf step length 19"() -> (w1006:dbl)
                n917 = local read "rf step length 20"() -> (w1013:dbl)
                n918 = local read "rf step length 17"() -> (w1009:dbl)
                n919 = local read "rf step length 18"() -> (w1005:dbl)
                n920 = local read "rf step length 16"() -> (w1010:dbl)
                n921 = local read "rf step length 14"() -> (w1001:dbl)
                n922 = local read "rf step length 12"() -> (w998:dbl)
                n923 = local read "rf step length 13"() -> (w1002:dbl)
                n924 = local read "rf step length 11"() -> (w997:dbl)
                n925 = local read "rf step length 15"() -> (w1014:dbl)
                n926 = Number To Decimal String(number=w1006) -> (decimal integer string=w1049:string)  [unwired: 1 in]
                n927 = Number To Decimal String(number=w1013) -> (decimal integer string=w1047:string)  [unwired: 1 in]
                n928 = Number To Decimal String(number=w1009) -> (decimal integer string=w1053:string)  [unwired: 1 in]
                n929 = Number To Decimal String(number=w1005) -> (decimal integer string=w1051:string)  [unwired: 1 in]
                n930 = Number To Decimal String(number=w1010) -> (decimal integer string=w1055:string)  [unwired: 1 in]
                n931 = Number To Decimal String(number=w1001) -> (decimal integer string=w1043:string)  [unwired: 1 in]
                n932 = Number To Decimal String(number=w998) -> (decimal integer string=w1039:string)  [unwired: 1 in]
                n933 = Number To Decimal String(number=w1002) -> (decimal integer string=w1041:string)  [unwired: 1 in]
                n934 = Number To Decimal String(number=w997) -> (decimal integer string=w1037:string)  [unwired: 1 in]
                n935 = Number To Decimal String(number=w1014) -> (decimal integer string=w1045:string)  [unwired: 1 in]
                n936 = Concatenate Strings("RF Step 19 length" ("string"), w1059, w1059, w1059, ":" ("string"), "\t", w1049, "\r\n") -> (w1024:string)
                n937 = Concatenate Strings("RF Step 20 length" ("string"), w1056, w1056, w1056, ":" ("string"), "\t", w1047, "\r\n") -> (w1025:string)
                n938 = Concatenate Strings("RF Step 17 length" ("string"), w1062, w1062, w1062, ":" ("string"), "\t", w1053, "\r\n") -> (w1022:string)
                n939 = Concatenate Strings("RF Step 18 length" ("string"), w1061, w1061, w1061, ":" ("string"), "\t", w1051, "\r\n") -> (w1023:string)
                n940 = Concatenate Strings("RF Step 16 length" ("string"), w1064, w1064, w1064, ":" ("string"), "\t", w1055, "\r\n") -> (w1021:string)
                n941 = Concatenate Strings("RF Step 14 length" ("string"), w1069, w1069, w1069, ":" ("string"), "\t", w1043, "\r\n") -> (w1019:string)
                n942 = Concatenate Strings("RF Step 15 length" ("string"), w1066, w1066, w1066, ":" ("string"), "\t", w1045, "\r\n") -> (w1020:string)
                n943 = Concatenate Strings("RF Step 12 length" ("string"), w1073, w1073, w1073, ":" ("string"), "\t", w1039, "\r\n") -> (w1017:string)
                n944 = Concatenate Strings("RF Step 13 length" ("string"), w1071, w1071, w1071, ":" ("string"), "\t", w1041, "\r\n") -> (w1018:string)
                n945 = Concatenate Strings("RF Step 11 length" ("string"), w1074, w1074, w1074, ":" ("string"), "\t", w1037, "\r\n") -> (w1016:string)
                n946 = Concatenate Strings(w1016, w1017, w1018, w1019, w1020) -> (w995:string)
                n947 = Concatenate Strings(w1021, w1022, w1023, w1024, w1025) -> (w993:string)
                n948 = Concatenate Strings(w995, w993, w992) -> (w994:string)
                n949 = Concatenate Strings(w1135, w1135, w1136, w1132, w994) -> (w1197:string)
                n950 = Concatenate Strings(w1134, w1197) -> (w1133:string)
              }
              frame #6 {
                n951 = local read "Recipe Name"() -> (w1203:string)
                n952 = call "File Dialog2"("start path"=path "D:/VK-1701 System Files/Recipe Files", "default name"=w1203) -> ("selected path"=w1201:path, "cancelled"=w1200:bool, "error out"=→"error out":errorcluster)  [unwired: 10 in, 1 out]
                n953 = case shown="True" w1200 {
                  tunnel: w1201 -> [w1213 _]
                  tunnel: [w1213 path "" ("selected path")] -> w1198
                  frame False {
                  }
                  frame True {
                  }
                }
                n954 = case shown="False" w1200 {
                  tunnel: w1199 -> [w1206 _]
                  tunnel: w1198 -> [w1205 _]
                  frame False {
                    n955 = Open/Create/Replace File(file path (use dialog)=w1205, operation (0:open)=T4."replace or create", access (0:read/write)=enum16{"read/write", "read-only", "write-only"}."read/write") -> (refnum out=w1208:refnum<file>, error out=w1207:errorcluster)  [unwired: 3 in, 1 out]
                    n956 = Write to Text File(file (use dialog)=w1208, text=w1206, error in=w1207) -> (refnum out=w1210:refnum<file>, error out=w1209:errorcluster)  [unwired: 1 in, 1 out]
                    n957 = Close File(refnum=w1210, error in=w1209) -> ()  [unwired: 2 out]
                  }
                  frame True {
                  }
                }
                "concatenated string" <- w1199
              }
              frame #7 {
              }
            }
          }
        }
        n958 = Equal?(x="flexmag", y="password") -> (x = y?=w337:bool)
        n959 = And(x=w337, y="password") -> (x .and. y?=w335:bool)
        n960 = case shown="True" w335 {
          frame False {
          }
          frame True {
            n961 = property on="hidden tab" class="TabCtl (strict)"("Visible"=TRUE) -> ()  [unwired: 2 in, 2 out]
            n962 = property on="concatenated string" class="Str"("Visible"=TRUE) -> ()  [unwired: 2 in, 2 out]
          }
        }
        n963 = local read "CANCEL"() -> (w341:bool)
        n964 = Or(x=w342, y=w341) -> (x .or. y?=w343:bool)
      }
      n965 = while {
        stop <- w24 stop-if-true
        n966 = local read "CANCEL"() -> (w26:bool)
        n967 = local read "done"() -> (w25:bool)
        n968 = Wait Until Next ms Multiple(millisecond multiple=u32 300) -> ()  [unwired: 1 out]
        n969 = case shown="True" "LOAD" {
          frame False {
          }
          frame True {
            n970 = stacked-sequence {
              frame #0 {
                n971 = call "File Dialog"("start path"=path "D:/VK-1701 System Files/Recipe Files") -> ("selected path"=w42:path, "cancelled"=w41:bool, "error out"=→"error out 2":errorcluster)  [unwired: 11 in, 1 out]
                n972 = case shown="False" w41 {
                  tunnel: [w203 string[][] [] ("all rows")] -> w201
                  tunnel: w42 -> [w202 _]
                  frame False {
                    n973 = call-poly <vilib>:"Read Delimited Spreadsheet.vi"("file path (dialog if empty)"=w202) -> ("all rows"=w203:string[][])  [unwired: 9 in, 5 out]
                  }
                  frame True {
                  }
                }
                n974 = Index Array(array=w201, index (row) #1=0 ("index (row)"), index (col) #1=4 ("index (row)"), index (row) #2=1 ("index (row)"), index (col) #2=4 ("index (row)"), index (row) #3=4 ("index (row)"), index (col) #3=4 ("index (row)"), index (row) #4=5 ("index (row)"), index (col) #4=4 ("index (row)"), index (row) #5=8 ("index (row)"), index (col) #5=4 ("index (row)"), index (row) #6=9 ("index (row)"), index (col) #6=4 ("index (row)"), index (row) #7=10 ("index (row)"), index (col) #7=4 ("index (row)"), index (row) #8=13 ("index (row)"), index (col) #8=4 ("index (row)"), index (row) #9=14 ("index (row)"), index (col) #9=4 ("index (row)"), index (row) #10=17 ("index (row)"), index (col) #10=4 ("index (row)"), index (row) #11=18 ("index (row)"), index (col) #11=4 ("index (row)"), index (row) #12=21 ("index (row)"), index (col) #12=4 ("index (row)"), index (row) #13=28 ("index (row)"), index (col) #13=4 ("index (row)"), index (row) #14=29 ("index (row)"), index (col) #14=4 ("index (row)"), index (row) #15=30 ("index (row)"), index (col) #15=4 ("index (row)"), index (row) #16=31 ("index (row)"), index (col) #16=4 ("index (row)"), index (row) #17=32 ("index (row)"), index (col) #17=4 ("index (row)"), index (row) #18=33 ("index (row)"), index (col) #18=4 ("index (row)"), index (row) #19=34 ("index (row)"), index (col) #19=4 ("index (row)"), index (row) #20=35 ("index (row)"), index (col) #20=4 ("index (row)"), index (row) #21=36 ("index (row)"), index (col) #21=4 ("index (row)"), index (row) #22=37 ("index (row)"), index (col) #22=4 ("index (row)"), index (row) #23=40 ("index (row)"), index (col) #23=4 ("index (row)"), index (row) #24=41 ("index (row)"), index (col) #24=4 ("index (row)"), index (row) #25=42 ("index (row)"), index (col) #25=4 ("index (row)"), index (row) #26=43 ("index (row)"), index (col) #26=4 ("index (row)"), index (row) #27=44 ("index (row)"), index (col) #27=4 ("index (row)"), index (row) #28=45 ("index (row)"), index (col) #28=4 ("index (row)"), index (row) #29=46 ("index (row)"), index (col) #29=4 ("index (row)"), index (row) #30=47 ("index (row)"), index (col) #30=4 ("index (row)"), index (row) #31=48 ("index (row)"), index (col) #31=4 ("index (row)"), index (row) #32=49 ("index (row)"), index (col) #32=4 ("index (row)"), index (row) #33=54 ("index (row)"), index (col) #33=4 ("index (row)"), index (row) #34=55 ("index (row)"), index (col) #34=4 ("index (row)"), index (row) #35=56 ("index (row)"), index (col) #35=4 ("index (row)"), index (row) #36=57 ("index (row)"), index (col) #36=4 ("index (row)"), index (row) #37=58 ("index (row)"), index (col) #37=4 ("index (row)"), index (row) #38=59 ("index (row)"), index (col) #38=4 ("index (row)"), index (row) #39=60 ("index (row)"), index (col) #39=4 ("index (row)"), index (row) #40=61 ("index (row)"), index (col) #40=4 ("index (row)"), index (row) #41=62 ("index (row)"), index (col) #41=4 ("index (row)"), index (row) #42=63 ("index (row)"), index (col) #42=4 ("index (row)"), index (row) #43=66 ("index (row)"), index (col) #43=4 ("index (row)"), index (row) #44=67 ("index (row)"), index (col) #44=4 ("index (row)"), index (row) #45=68 ("index (row)"), index (col) #45=4 ("index (row)"), index (row) #46=69 ("index (row)"), index (col) #46=4 ("index (row)"), index (row) #47=70 ("index (row)"), index (col) #47=4 ("index (row)"), index (row) #48=71 ("index (row)"), index (col) #48=4 ("index (row)"), index (row) #49=72 ("index (row)"), index (col) #49=4 ("index (row)"), index (row) #50=73 ("index (row)"), index (col) #50=4 ("index (row)"), index (row) #51=74 ("index (row)"), index (col) #51=4 ("index (row)"), index (row) #52=75 ("index (row)"), index (col) #52=4 ("index (row)"), index (row) #53=78 ("index (row)"), index (col) #53=4 ("index (row)"), index (row) #54=79 ("index (row)"), index (col) #54=4 ("index (row)"), index (row) #55=82 ("index (row)"), index (col) #55=4 ("index (row)"), index (row) #56=83 ("index (row)"), index (col) #56=4 ("index (row)")) -> (element #1=→"L recipe name":string, element #2=→"L sbs name":string, element #3=→"L recipe selection":string, element #4=→"L web selection":string, element #5=→"L core diamater":string, element #6=→"L left init diamater":string, element #7=→"L web thickness":string, element #8=→"L web speed":string, element #9=→"L tension  value":string, element #10=→"L single process type selection":string, element #11=→"L chamber selection":string, element #12=→"L microwave power":string, element #13=→"L dc power step 1":string, element #14=→"L dc power step 2":string, element #15=→"L dc power step 3":string, element #16=→"L dc power step 4":string, element #17=→"L dc power step 5":string, element #18=→"L dc power step 6":string, element #19=→"L dc power step 7":string, element #20=→"L dc power step 8":string, element #21=→"L dc power step 9":string, element #22=→"L dc power step 10":string, element #23=→"L dc length step 1":string, element #24=→"L dc length step 2":string, element #25=→"L dc length step 3":string, element #26=→"L dc length step 4":string, element #27=→"L dc length step 5":string, element #28=→"L dc length step 6":string, element #29=→"L dc length step 7":string, element #30=→"L dc length step 8":string, element #31=→"L dc length step 9":string, element #32=→"L dc length step 10":string, element #33=→"L rf power step 1":string, element #34=→"L rf power step 2":string, element #35=→"L rf power step 3":string, element #36=→"L rf power step 4":string, element #37=→"L rf power step 5":string, element #38=→"L rf power step 6":string, element #39=→"L rf power step 7":string, element #40=→"L rf power step 8":string, element #41=→"L rf power step 9":string, element #42=→"L rf power step 10":string, element #43=→"L rf length step 1":string, element #44=→"L rf length step 2":string, element #45=→"L rf length step 3":string, element #46=→"L rf length step 4":string, element #47=→"L rf length step 5":string, element #48=→"L rf length step 6":string, element #49=→"L rf length step 7":string, element #50=→"L rf length step 8":string, element #51=→"L rf length step 9":string, element #52=→"L rf length step 10":string, element #53=→"L argon flow":string, element #54=→"L pressure":string, element #55=→"L rf step number":string, element #56=→"L dc step number":string)
              }
              frame #1 {
                n975 = local read "L dc power step 10"() -> (w274:string)
                n976 = local read "L dc power step 9"() -> (w281:string)
                n977 = local read "L dc power step 8"() -> (w280:string)
                n978 = local read "L dc power step 1"() -> (w298:string)
                n979 = local read "L dc power step 7"() -> (w276:string)
                n980 = local read "L dc power step 2"() -> (w299:string)
                n981 = local read "L dc power step 4"() -> (w284:string)
                n982 = local read "L dc power step 3"() -> (w285:string)
                n983 = local read "L dc power step 5"() -> (w271:string)
                n984 = local read "L dc power step 6"() -> (w277:string)
                n985 = local read "L recipe selection"() -> (w319:string)
                n986 = local read "L web selection"() -> (w315:string)
                n987 = local read "L recipe name"() -> (w321:string)
                n988 = local read "L sbs name"() -> (w320:string)
                n989 = Decimal String To Number(string=w274) -> (number=w273:i32)  [unwired: 2 in, 1 out]
                n990 = Decimal String To Number(string=w281) -> (number=w282:i32)  [unwired: 2 in, 1 out]
                n991 = Decimal String To Number(string=w280) -> (number=w279:i32)  [unwired: 2 in, 1 out]
                n992 = Decimal String To Number(string=w298) -> (number=w297:i32)  [unwired: 2 in, 1 out]
                n993 = Decimal String To Number(string=w276) -> (number=w275:i32)  [unwired: 2 in, 1 out]
                n994 = Decimal String To Number(string=w299) -> (number=w300:i32)  [unwired: 2 in, 1 out]
                n995 = Decimal String To Number(string=w284) -> (number=w283:i32)  [unwired: 2 in, 1 out]
                n996 = Decimal String To Number(string=w285) -> (number=w286:i32)  [unwired: 2 in, 1 out]
                n997 = Decimal String To Number(string=w271) -> (number=w272:i32)  [unwired: 2 in, 1 out]
                n998 = Decimal String To Number(string=w277) -> (number=w278:i32)  [unwired: 2 in, 1 out]
                n999 = Equal?(x=w315, y="Web") -> (x = y?=w313:bool)
                n1000 = Equal?(x=w319, y="Single Recipe") -> (x = y?=w317:bool)
                n1001 = local write "dc step watt 10"(w273) -> ()
                n1002 = local write "dc step watt 9"(w282) -> ()
                n1003 = local write "dc step watt 1"(w297) -> ()
                n1004 = local write "dc step watt 8"(w279) -> ()
                n1005 = local write "dc step watt 7"(w275) -> ()
                n1006 = local write "dc step watt 2"(w300) -> ()
                n1007 = local write "dc step watt 4"(w283) -> ()
                n1008 = local write "dc step watt 3"(w286) -> ()
                n1009 = local write "dc step watt 5"(w272) -> ()
                n1010 = local write "dc step watt 6"(w278) -> ()
                n1011 = case shown="True" w317 {
                  tunnel: [w333 w334] -> w316
                  frame False {
                    w333 = u16 1 items=["single recipe", "multilayer recipe"] ("Recipe Selection")
                  }
                  frame True {
                    w334 = u16 0 items=["single recipe", "multilayer recipe"] ("Recipe Selection")
                  }
                }
                n1012 = case shown="False" w313 {
                  tunnel: [w331 w332] -> w312
                  frame False {
                    w331 = u16 1 items=["web", "other"] ("Web Selection")
                  }
                  frame True {
                    w332 = u16 0 items=["web", "other"] ("Web Selection")
                  }
                }
                n1013 = local write "Substrate Material"(w320) -> ()
                n1014 = local write "Recipe Name"(w321) -> ()
                n1015 = local read "L dc length step 1"() -> (w253:string)
                n1016 = local read "L dc length step 10"() -> (w267:string)
                n1017 = local read "L dc length step 7"() -> (w265:string)
                n1018 = local read "L dc length step 2"() -> (w252:string)
                n1019 = local read "L dc length step 4"() -> (w257:string)
                n1020 = local read "L dc length step 9"() -> (w260:string)
                n1021 = local read "L dc length step 3"() -> (w256:string)
                n1022 = local read "L dc length step 5"() -> (w270:string)
                n1023 = local read "L dc length step 6"() -> (w264:string)
                n1024 = local read "L dc length step 8"() -> (w261:string)
                n1025 = local write "Recipe Selection"(w316) -> ()
                n1026 = local write "Web Selection"(w312) -> ()
                n1027 = Wait (ms)(milliseconds to wait=u32 100) -> ()  [unwired: 1 out]
                n1028 = Decimal String To Number(string=w253) -> (number=w254:i32)  [unwired: 2 in, 1 out]
                n1029 = Decimal String To Number(string=w265) -> (number=w266:i32)  [unwired: 2 in, 1 out]
                n1030 = Decimal String To Number(string=w252) -> (number=w251:i32)  [unwired: 2 in, 1 out]
                n1031 = Decimal String To Number(string=w257) -> (number=w258:i32)  [unwired: 2 in, 1 out]
                n1032 = Decimal String To Number(string=w260) -> (number=w259:i32)  [unwired: 2 in, 1 out]
                n1033 = Decimal String To Number(string=w267) -> (number=w268:i32)  [unwired: 2 in, 1 out]
                n1034 = Decimal String To Number(string=w256) -> (number=w255:i32)  [unwired: 2 in, 1 out]
                n1035 = Decimal String To Number(string=w270) -> (number=w269:i32)  [unwired: 2 in, 1 out]
                n1036 = Decimal String To Number(string=w264) -> (number=w263:i32)  [unwired: 2 in, 1 out]
                n1037 = Decimal String To Number(string=w261) -> (number=w262:i32)  [unwired: 2 in, 1 out]
                n1038 = local write "dc step length 1"(w254) -> ()
                n1039 = local write "dc step length 10"(w268) -> ()
                n1040 = local write "dc step length 7"(w266) -> ()
                n1041 = local write "dc step length 2"(w251) -> ()
                n1042 = local write "dc step length 4"(w258) -> ()
                n1043 = local write "dc step length 9"(w259) -> ()
                n1044 = local write "dc step length 3"(w255) -> ()
                n1045 = local write "dc step length 5"(w269) -> ()
                n1046 = local write "dc step length 6"(w263) -> ()
                n1047 = local write "dc step length 8"(w262) -> ()
                n1048 = local read "L microwave power"() -> (w295:string)
                n1049 = local read "L left init diamater"() -> (w310:string)
                n1050 = local read "L core diamater"() -> (w311:string)
                n1051 = local read "L web thickness"() -> (w305:string)
                n1052 = local read "L tension  value"() -> (w301:string)
                n1053 = local read "L web speed"() -> (w304:string)
                n1054 = Decimal String To Number(string=w295) -> (number=w296:i32)  [unwired: 2 in, 1 out]
                n1055 = Decimal String To Number(string=w311) -> (number=w309:i32)  [unwired: 2 in, 1 out]
                n1056 = Decimal String To Number(string=w305) -> (number=w306:i32)  [unwired: 2 in, 1 out]
                n1057 = Decimal String To Number(string=w301) -> (number=w302:i32)  [unwired: 2 in, 1 out]
                n1058 = Decimal String To Number(string=w304) -> (number=w303:i32)  [unwired: 2 in, 1 out]
                n1059 = Fract/Exp String To Number(use system decimal point (T)=FALSE, string=w310) -> (number=w308:dbl)  [unwired: 2 in, 1 out]
                n1060 = local write "power microwave"(w296) -> ()
                n1061 = local write "left initial diameter"(w308) -> ()
                n1062 = local write "core diameter"(w309) -> ()
                n1063 = local write "web thickness"(w306) -> ()
                n1064 = local write "tension value"(w302) -> ()
                n1065 = local write "web speed"(w303) -> ()
                n1066 = local read "L rf power step 10"() -> (w227:string)
                n1067 = local read "L rf power step 9"() -> (w220:string)
                n1068 = local read "L rf power step 8"() -> (w221:string)
                n1069 = local read "L rf power step 1"() -> (w213:string)
                n1070 = local read "L rf power step 7"() -> (w225:string)
                n1071 = local read "L dc power step 6"() -> (w224:string)
                n1072 = local read "L rf power step 2"() -> (w212:string)
                n1073 = local read "L rf power step 4"() -> (w217:string)
                n1074 = local read "L rf power step 3"() -> (w216:string)
                n1075 = local read "L rf power step 5"() -> (w230:string)
                n1076 = Decimal String To Number(string=w227) -> (number=w228:i32)  [unwired: 2 in, 1 out]
                n1077 = local read "L single process type selection"() -> (w294:string)
                n1078 = Decimal String To Number(string=w220) -> (number=w219:i32)  [unwired: 2 in, 1 out]
                n1079 = Decimal String To Number(string=w221) -> (number=w222:i32)  [unwired: 2 in, 1 out]
                n1080 = Decimal String To Number(string=w213) -> (number=w214:i32)  [unwired: 2 in, 1 out]
                n1081 = Decimal String To Number(string=w225) -> (number=w226:i32)  [unwired: 2 in, 1 out]
                n1082 = Decimal String To Number(string=w212) -> (number=w211:i32)  [unwired: 2 in, 1 out]
                n1083 = Decimal String To Number(string=w217) -> (number=w218:i32)  [unwired: 2 in, 1 out]
                n1084 = Decimal String To Number(string=w216) -> (number=w215:i32)  [unwired: 2 in, 1 out]
                n1085 = Decimal String To Number(string=w230) -> (number=w229:i32)  [unwired: 2 in, 1 out]
                n1086 = Decimal String To Number(string=w224) -> (number=w223:i32)  [unwired: 2 in, 1 out]
                n1087 = local read "L chamber selection"() -> (w290:string)
                n1088 = local write "rf step watt 10"(w228) -> ()
                n1089 = local write "rf step watt 9"(w219) -> ()
                n1090 = local write "rf step watt 8"(w222) -> ()
                n1091 = local write "rf step watt 1"(w214) -> ()
                n1092 = local write "rf step watt 7"(w226) -> ()
                n1093 = local write "rf step watt 2"(w211) -> ()
                n1094 = local write "rf step watt 4"(w218) -> ()
                n1095 = local write "rf step watt 3"(w215) -> ()
                n1096 = local write "rf step watt 5"(w229) -> ()
                n1097 = local write "rf step watt 6"(w223) -> ()
                n1098 = Equal?(x=w290, y="III" ("L single process")) -> (x = y?=w288:bool)
                n1099 = Equal?(x=w294, y="Microwave" ("L single process")) -> (x = y?=w292:bool)
                n1100 = case shown="True" w292 {
                  tunnel: [w324 enum32{"microwave", "dcsputter", "rfsputter"}."microwave" ("single process selection")] -> w291
                  frame False {
                    n1101 = local read "L single process type selection"() -> (w326:string)
                    n1102 = Equal?(x=w326, y="RF Sputter" ("L single process")) -> (x = y?=w325:bool)
                    n1103 = case shown="False" w325 {
                      tunnel: [enum32{"microwave", "dcsputter", "rfsputter"}."dcsputter" ("single process selection") enum32{"microwave", "dcsputter", "rfsputter"}."rfsputter" ("single process selection")] -> w324
                      frame False {
                      }
                      frame True {
                      }
                    }
                  }
                  frame True {
                  }
                }
                n1104 = case shown="False" w288 {
                  tunnel: [enum32{"chamber II", "chamber III"}."chamber II" ("DC Sputter Chamber Selection") enum32{"chamber II", "chamber III"}."chamber III" ("DC Sputter Chamber Selection")] -> w287
                  frame False {
                  }
                  frame True {
                  }
                }
                n1105 = local read "L pressure"() -> (w207:string)
                n1106 = local read "L rf length step 1"() -> (w248:string)
                n1107 = local read "L rf length step 10"() -> (w234:string)
                n1108 = local read "L argon flow"() -> (w205:string)
                n1109 = local read "L rf length step 7"() -> (w236:string)
                n1110 = local read "L rf length step 2"() -> (w249:string)
                n1111 = local read "L rf length step 4"() -> (w244:string)
                n1112 = local read "L rf length step 9"() -> (w241:string)
                n1113 = local read "L rf length step 3"() -> (w245:string)
                n1114 = local read "L rf length step 5"() -> (w231:string)
                n1115 = local read "L rf length step 6"() -> (w237:string)
                n1116 = local read "L rf length step 8"() -> (w240:string)
                n1117 = Fract/Exp String To Number(use system decimal point (T)=FALSE, string=w207) -> (number=w208:dbl)  [unwired: 2 in, 1 out]
                n1118 = Decimal String To Number(string=w205) -> (number=w206:i32)  [unwired: 2 in, 1 out]
                n1119 = Decimal String To Number(string=w248) -> (number=w247:i32)  [unwired: 2 in, 1 out]
                n1120 = Decimal String To Number(string=w236) -> (number=w235:i32)  [unwired: 2 in, 1 out]
                n1121 = Decimal String To Number(string=w249) -> (number=w250:i32)  [unwired: 2 in, 1 out]
                n1122 = Decimal String To Number(string=w244) -> (number=w243:i32)  [unwired: 2 in, 1 out]
                n1123 = Decimal String To Number(string=w241) -> (number=w242:i32)  [unwired: 2 in, 1 out]
                n1124 = Decimal String To Number(string=w234) -> (number=w233:i32)  [unwired: 2 in, 1 out]
                n1125 = Decimal String To Number(string=w245) -> (number=w246:i32)  [unwired: 2 in, 1 out]
                n1126 = Decimal String To Number(string=w231) -> (number=w232:i32)  [unwired: 2 in, 1 out]
                n1127 = Decimal String To Number(string=w237) -> (number=w238:i32)  [unwired: 2 in, 1 out]
                n1128 = Decimal String To Number(string=w240) -> (number=w239:i32)  [unwired: 2 in, 1 out]
                n1129 = local write "DC Sputter Chamber Selection"(w287) -> ()
                n1130 = local write "Pressure set mbar"(w208) -> ()
                n1131 = local write "Ar set sccm"(w206) -> ()
                n1132 = local write "rf step length 1"(w247) -> ()
                n1133 = local write "rf step length 10"(w233) -> ()
                n1134 = local write "rf step length 7"(w235) -> ()
                n1135 = local write "rf step length 2"(w250) -> ()
                n1136 = local write "rf step length 4"(w243) -> ()
                n1137 = local write "rf step length 9"(w242) -> ()
                n1138 = local write "rf step length 3"(w246) -> ()
                n1139 = local write "rf step length 5"(w232) -> ()
                n1140 = local write "rf step length 6"(w238) -> ()
                n1141 = local write "rf step length 8"(w239) -> ()
                n1142 = local write "single process selection"(w291) -> ()
              }
            }
          }
        }
        n1143 = Or(x=w25, y=w26) -> (x .or. y?=w24:bool)
      }
    }
  }
